vi "MainPannel.vi"() -> ()   [LabVIEW 2018]
uses:
  Controls/StageInfo.ctl
  Controls/GeneratorInfo.ctl
  <vilib>/userdefined/High Color/nirio_resource_hc.ctl
  Controls/DigitizerInfo.ctl
  Controls/AdditionalData.ctl
  <vilib>/Heliosphere Research LLC/Advanced Plotting Toolkit/properties/Colormap_Map.ctl
  <vilib>/Math Plots/3D Math Plots/3D Mesh/3D Mesh XCtrl/3D Mesh.xctl
  Controls/ScanStates.ctl
  Program_Files/Labview2018/MAIN/instr.lib/ASI TG-1000/Public/Utility/Axis Name.ctl
  <vilib>/UPVI/lvhdf5/dataset.llb/LVH5D Operation.ctl
  <extravilib>/ChannelInstances/Tag-c(t'AdditionalData.ctl',bool)/Write With Abort.vi
  <extravilib>/ChannelInstances/Tag-c(t'GeneratorInfo.ctl',bool)/Write With Abort.vi
  <extravilib>/ChannelInstances/Tag-c(t'DigitizerInfo.ctl',bool)/Write With Abort.vi
  <extravilib>/ChannelInstances/Tag-c(t'StageInfo.ctl',bool)/Write With Abort.vi
  <extravilib>/ChannelInstances/Tag-c(t'AdditionalData.ctl',bool)/Read With Abort.vi
  <extravilib>/ChannelInstances/Tag-c(t'GeneratorInfo.ctl',bool)/Read With Abort.vi
  <extravilib>/ChannelInstances/Tag-c(t'DigitizerInfo.ctl',bool)/Read With Abort.vi
  <extravilib>/ChannelInstances/Tag-c(t'StageInfo.ctl',bool)/Read With Abort.vi
  <extravilib>/ChannelInstances/Stream-c(i32,i32,a[.](u64))/Read With Abort.vi
  <extravilib>/ChannelInstances/Stream-c(i32,i32,a[.](u64))/Write With Abort.vi
  <extravilib>/ChannelInstances/Stream-c(i32,i32,a[.](u64))/EndpointRead.vi
  <extravilib>/ChannelInstances/Stream-c(i32,i32,a[.](u64))/Endpoint.vi
  <extravilib>/ChannelInstances/Tag-c(t'DigitizerInfo.ctl',bool)/Instantiate.vi
  <extravilib>/ChannelInstances/Tag-c(t'DigitizerInfo.ctl',bool)/Endpoint.vi
  <extravilib>/ChannelInstances/Tag-c(t'GeneratorInfo.ctl',bool)/Instantiate.vi
  <extravilib>/ChannelInstances/Tag-c(t'GeneratorInfo.ctl',bool)/Endpoint.vi
  <extravilib>/ChannelInstances/Tag-c(t'AdditionalData.ctl',bool)/Instantiate.vi
  <extravilib>/ChannelInstances/Tag-c(t'AdditionalData.ctl',bool)/Endpoint.vi
  <extravilib>/ChannelInstances/Tag-c(t'StageInfo.ctl',bool)/Instantiate.vi
  <extravilib>/ChannelInstances/Tag-c(t'AdditionalData.ctl',bool)/EndpointRead.vi
  <extravilib>/ChannelInstances/Tag-c(t'GeneratorInfo.ctl',bool)/EndpointRead.vi
  <extravilib>/ChannelInstances/Tag-c(t'DigitizerInfo.ctl',bool)/EndpointRead.vi
  <extravilib>/ChannelInstances/Tag-c(t'StageInfo.ctl',bool)/EndpointRead.vi
  <vilib>/UPVI/lvhdf5/dataset.llb/Simple OpenCreateReplace Dataset (Variant).vi
  <extravilib>/ChannelInstances/Stream-c(i32,i32,a[.](u64))/Instantiate.vi
  <extravilib>/ChannelInstances/Stream-c(i32,i32,a[.](u64))/)Channel.vi
  <resource>/ChannelSupport/_ChannelSupport/WaitIfNeeded.vi
  <vilib>/UPVI/lvhdf5/dataset.llb/Append Element(s) to Dataset (Variant).vi
  <vilib>/Math Plots/3D Math Plots/3D Mesh/3D Mesh Datatype/Public/Plot Helper (Vector).vi
  <vilib>/Utility/error.llb/Error Cluster From Error Code.vi
  <vilib>/rvi/errors/niLvFpgaAdjustHostInterfaceError.vi
  <vilib>/FPGAPlugInAG/Dynamic/niLvFpga_Close_Dynamic.vi
  <extravilib>/ChannelInstances/Tag-c(t'StageInfo.ctl',bool)/Endpoint.vi
  <vilib>/UPVI/lvhdf5/dataset.llb/Simple OpenCreateReplace Dataset.xnode
  <vilib>/UPVI/lvhdf5/library.llb/HDF5 Ref.ctl
  <vilib>/UPVI/lvhdf5/dataset.llb/Append Element(s) to Dataset.xnode
  <vilib>/rvi/interface/nirviReadWriteControl/nirviReadWriteControl.xnode
  <vilib>/rvi/interface/nirviCloseFPGA/nirviCloseFPGA.xnode
  <vilib>/rvi/interface/nirviMethod/nirviMethod.xnode
  Program_Files/Labview2018/MAIN/instr.lib/ASI TG-1000/ASI TG-1000.lvlib
  <vilib>/Analysis/NI_AALPro.lvlib
  <vilib>/Math Plots/3D Math Plots/3D Mesh/3D Mesh Datatype/3D Mesh Datatype.lvclass
  <extravilib>/ChannelInstances/Tag-c(t'StageInfo.ctl',bool).lvlib
  <extravilib>/ChannelInstances/Tag-c(t'DigitizerInfo.ctl',bool).lvlib
  <extravilib>/ChannelInstances/Tag-c(t'GeneratorInfo.ctl',bool).lvlib
  <extravilib>/ChannelInstances/Tag-c(t'AdditionalData.ctl',bool).lvlib
  NiFpgaLv.dll
  <vilib>/rvi/interface/Simulation/niFpgaSimulationCallBeginRW.vi
  <vilib>/FPGAPlugInAG/Dynamic/niLvFpga_ReadFifo_Dynamic.vi
  <vilib>/rvi/errors/niLvFpgaMergeErrorWithErrorCode.vi
  <extravilib>/ChannelInstances/Stream-c(i32,i32,a[.](u64)).lvlib
  <vilib>/Heliosphere Research LLC/Advanced Plotting Toolkit/Advanced Plotting Toolkit.lvlib
panel:
  in  "Find Delay after Trig":bool
  in  "Threshold Magnitude":dbl
  out "State":T1
  in  "Setup Scan":bool
  out "Stage Set":bool
  out "Additional Data Set?":bool
  out "3D Mesh":refnum<class "3D Plot Datatype.lvclass">[](xcontrol)
  in  "Data Gating":bool
  in  "Colorbar":bool
  in  "Axis":bool
  in  "Colormap":T2
  out "Image":picture
  in  "Emergercy Stop":bool
  in  "Length":dbl
  in  "Start Depth":dbl
  in  "Pixel/mm":bool=TRUE caption="Mode"
  in  "Z Position":dbl
  in  "Y Position":dbl
  in  "X Position":dbl
  out "Stage Position":cluster{dbl[], dbl[]}(graph) caption="XY Graph - Dark"
  in  "Waveform Tab Control":T3(tab)
  out "Input Graph":cluster{"tv":dbl[], "DAC Codes":u16[]}(graph)
  out "Output Graph":cluster{dbl, dbl, ext[][]}(graph)
  out "Output Graph FFT":cluster{dbl[], dbl[]}(graph)
  out "Additional Info":T4
  in  "Setup Additional Data":bool
  out "Digitizer Info":T5
  out "Default Configured?":bool
  out "Clocking Option Configured?":bool
  out "TIS Configured?":bool
  in  "Setup Digitizer":bool
  out "Generator Info":T7
  out "Stage Setup Info":T8
  in  "Setup Generator":bool
  in  "Setup Stage":bool
  in  "Update Stage Pos":bool
  out "Digitizer Configured?":bool
  out "Generator Ready?":bool
  out "Total Pixels":i32
  out "Stage Setup?":bool
  out "Scan Time":dbl
  out "Y Resolution":dbl
  out "X Resolution":dbl
  in  "Stage Control":T9(tab)
  in  "Stage Port":refnum<visa-resource-name>
  in  "Scan Mode":enum16{"Raster Scan", "Serpentine Scan"}(ring)
  in  "Start X":dbl
  in  "Start Y":dbl
  in  "Stop X":dbl=5.0 caption="X Length (mm)"
  in  "Stop Y":dbl=5.0 caption="Y Length (mm)"
  in  "Overshoot":dbl=1.0
  in  "X Speed (mms)":dbl=1.0
  in  "Y Speed (mms)":dbl=1.0
  in  "X Pixels Count":i32=40
  in  "Y Lines Count":i32=10
  in  "Use Current Position as Start":bool=TRUE caption="Checkbox"
  in  "Generator ID":tag
  in  "Digitizer ID":tag
  in  "Record Size (Samples)":u32=1024
  in  "Delay after Trigger (us)":dbl
  in  "Sampling Rate (Fs)":dbl=400000000.0 format="%#_6p"
  in  "Temperature":dbl
  in  "Trigger Type":enum8{"Software", "Data Edge"}(ring)
  in  "Trigger Level (V)":dbl
  in  "File Directory":path
  in  "Filename":string
  in  "Open Stage Port":bool
  in  "Move Z":i16(knob) scale=0.0..50.0
  in  "Move Y":i16(knob) scale=0.0..50.0
  in  "Move X":i16(knob) scale=0.0..50.0
  in  "Precision":i16(slide) scale=0.0..3.0
  in  "SendCommand To Stage":bool
  in  "Debug Mode":bool
  out "Response":string
  in  "Command":string
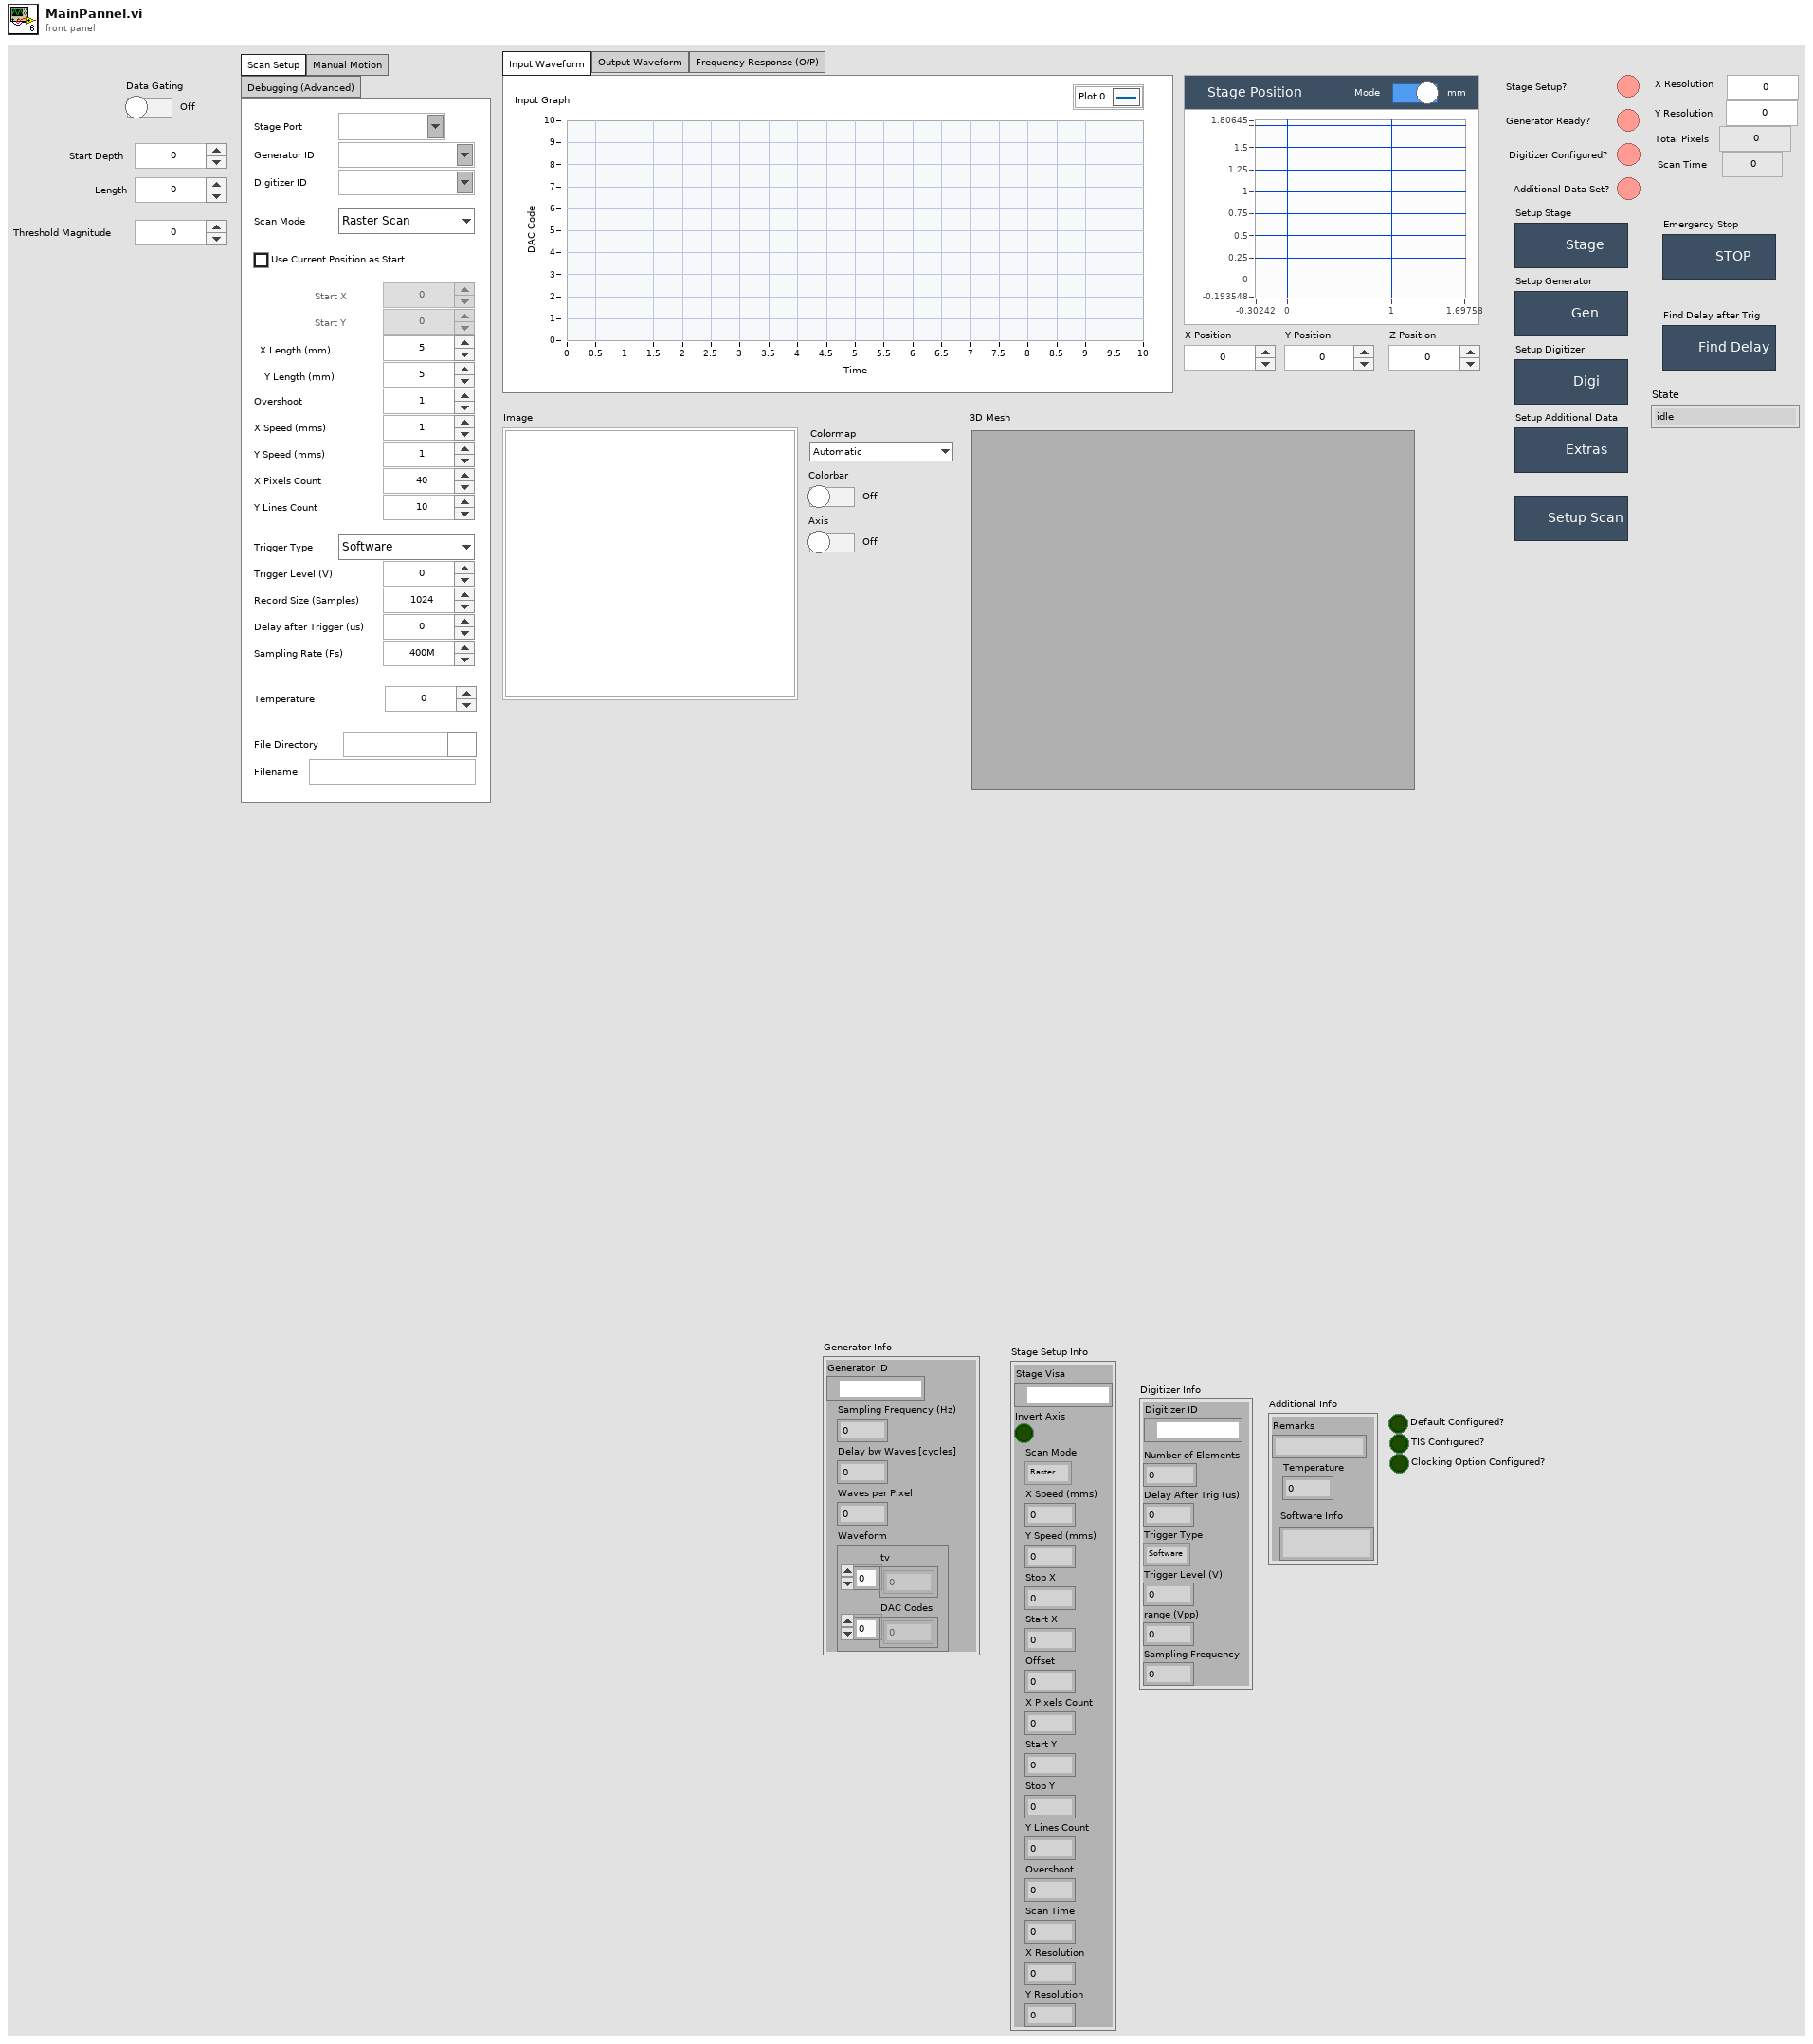
[diagram p1: front panel]
types:
  T1 = typedef "ScanStates.ctl" = enum16{"idle", "init", "scan", "endscan", "closefiles"}
  T2 = typedef "Advanced Plotting Toolkit.lvlib/Colormap_Map.ctl" = enum16{"Automatic", "Rainbow", "Hot and Cold", "White-Black", "White-Blue", "White-Green", "White-Red", "Fire", "Water", "Earth", "Air", "Pastel", "Banded", "Stepped"}
  T3 = enum32{"Input Waveform", "Output Waveform", "Frequency Response (O/P)"}
  T4 = typedef "AdditionalData.ctl" = cluster{"Remarks":string, "Temperature":dbl, "Software Info":string}
  T5 = typedef "DigitizerInfo.ctl" = cluster{"Digitizer ID":T6, "Number of Elements":u16, "Delay After Trig (us)":dbl, "Trigger Type":enum8{"Software", "Data Edge"}, "Trigger Level (V)":dbl, "range (Vpp)":dbl, "Sampling Frequency":dbl}
  T6 = typedef "nirio_resource_hc.ctl" = tag
  T7 = typedef "GeneratorInfo.ctl" = cluster{"Generator ID":T6, "Sampling Frequency (Hz)":u64, "Delay bw Waves [cycles]":u16, "Waves per Pixel":u32, "Waveform":cluster{"tv":dbl[], "DAC Codes":u16[]}}
  T8 = typedef "StageInfo.ctl" = cluster{"Stage Visa":refnum<visa-resource-name>, "Invert Axis":bool, "Scan Mode":enum16{"Raster Scan", "Serpentine Scan"}, "X Speed (mms)":dbl, "Y Speed (mms)":dbl, "Stop X":dbl, "Start X":dbl, "Offset":dbl, "X Pixels Count":i32, "Start Y":dbl, "Stop Y":dbl, "Y Lines Count":i32, "Overshoot":dbl, "Scan Time":dbl, "X Resolution":dbl, "Y Resolution":dbl}
  T9 = enum32{"Scan Setup", "Manual Motion", "Debugging (Advanced)"}
  T10 = enum8{"Enabled", "Disabled", "Disabled and Grayed Out"}
  T11 = typedef "Tag-c(t'StageInfo.ctl',bool).lvlib/))Channel.ctl" = refnum<queue>
  T12 = typedef "ASI TG-1000.lvlib/Axis Name.ctl" = enum8{"undefined", "A", "B", "C", "D", "E", "F", "G", "H", "I", "J", "K", "L", "M", "N", "O", "P", "Q", "R", "S", "T", "U", "V", "W", "X", "Y", "Z"}
  T13 = cluster{"Additional Info":T4, "Additional Data Set?":bool}
  T14 = typedef "Tag-c(t'AdditionalData.ctl',bool).lvlib/))Channel.ctl" = refnum<queue>
  T15 = typedef "Tag-c(t'GeneratorInfo.ctl',bool).lvlib/))Channel.ctl" = refnum<queue>
  T16 = typedef "Tag-c(t'DigitizerInfo.ctl',bool).lvlib/))Channel.ctl" = refnum<queue>
  T17 = typedef "LVH5D Operation.ctl" = enum16{"open", "replace", "create", "open or create", "create or replace", "create or replace with confirmation"}
  T18 = typedef "HDF5 Ref.ctl" = refnum<k1>
  T19 = typedef "Stream-c(i32,i32,a[.](u64)).lvlib/)Channel.ctl" = refnum<queue>
  T20 = cluster{"X Pixel":i32, "Y Pixel":i32, "Data":u64[]}
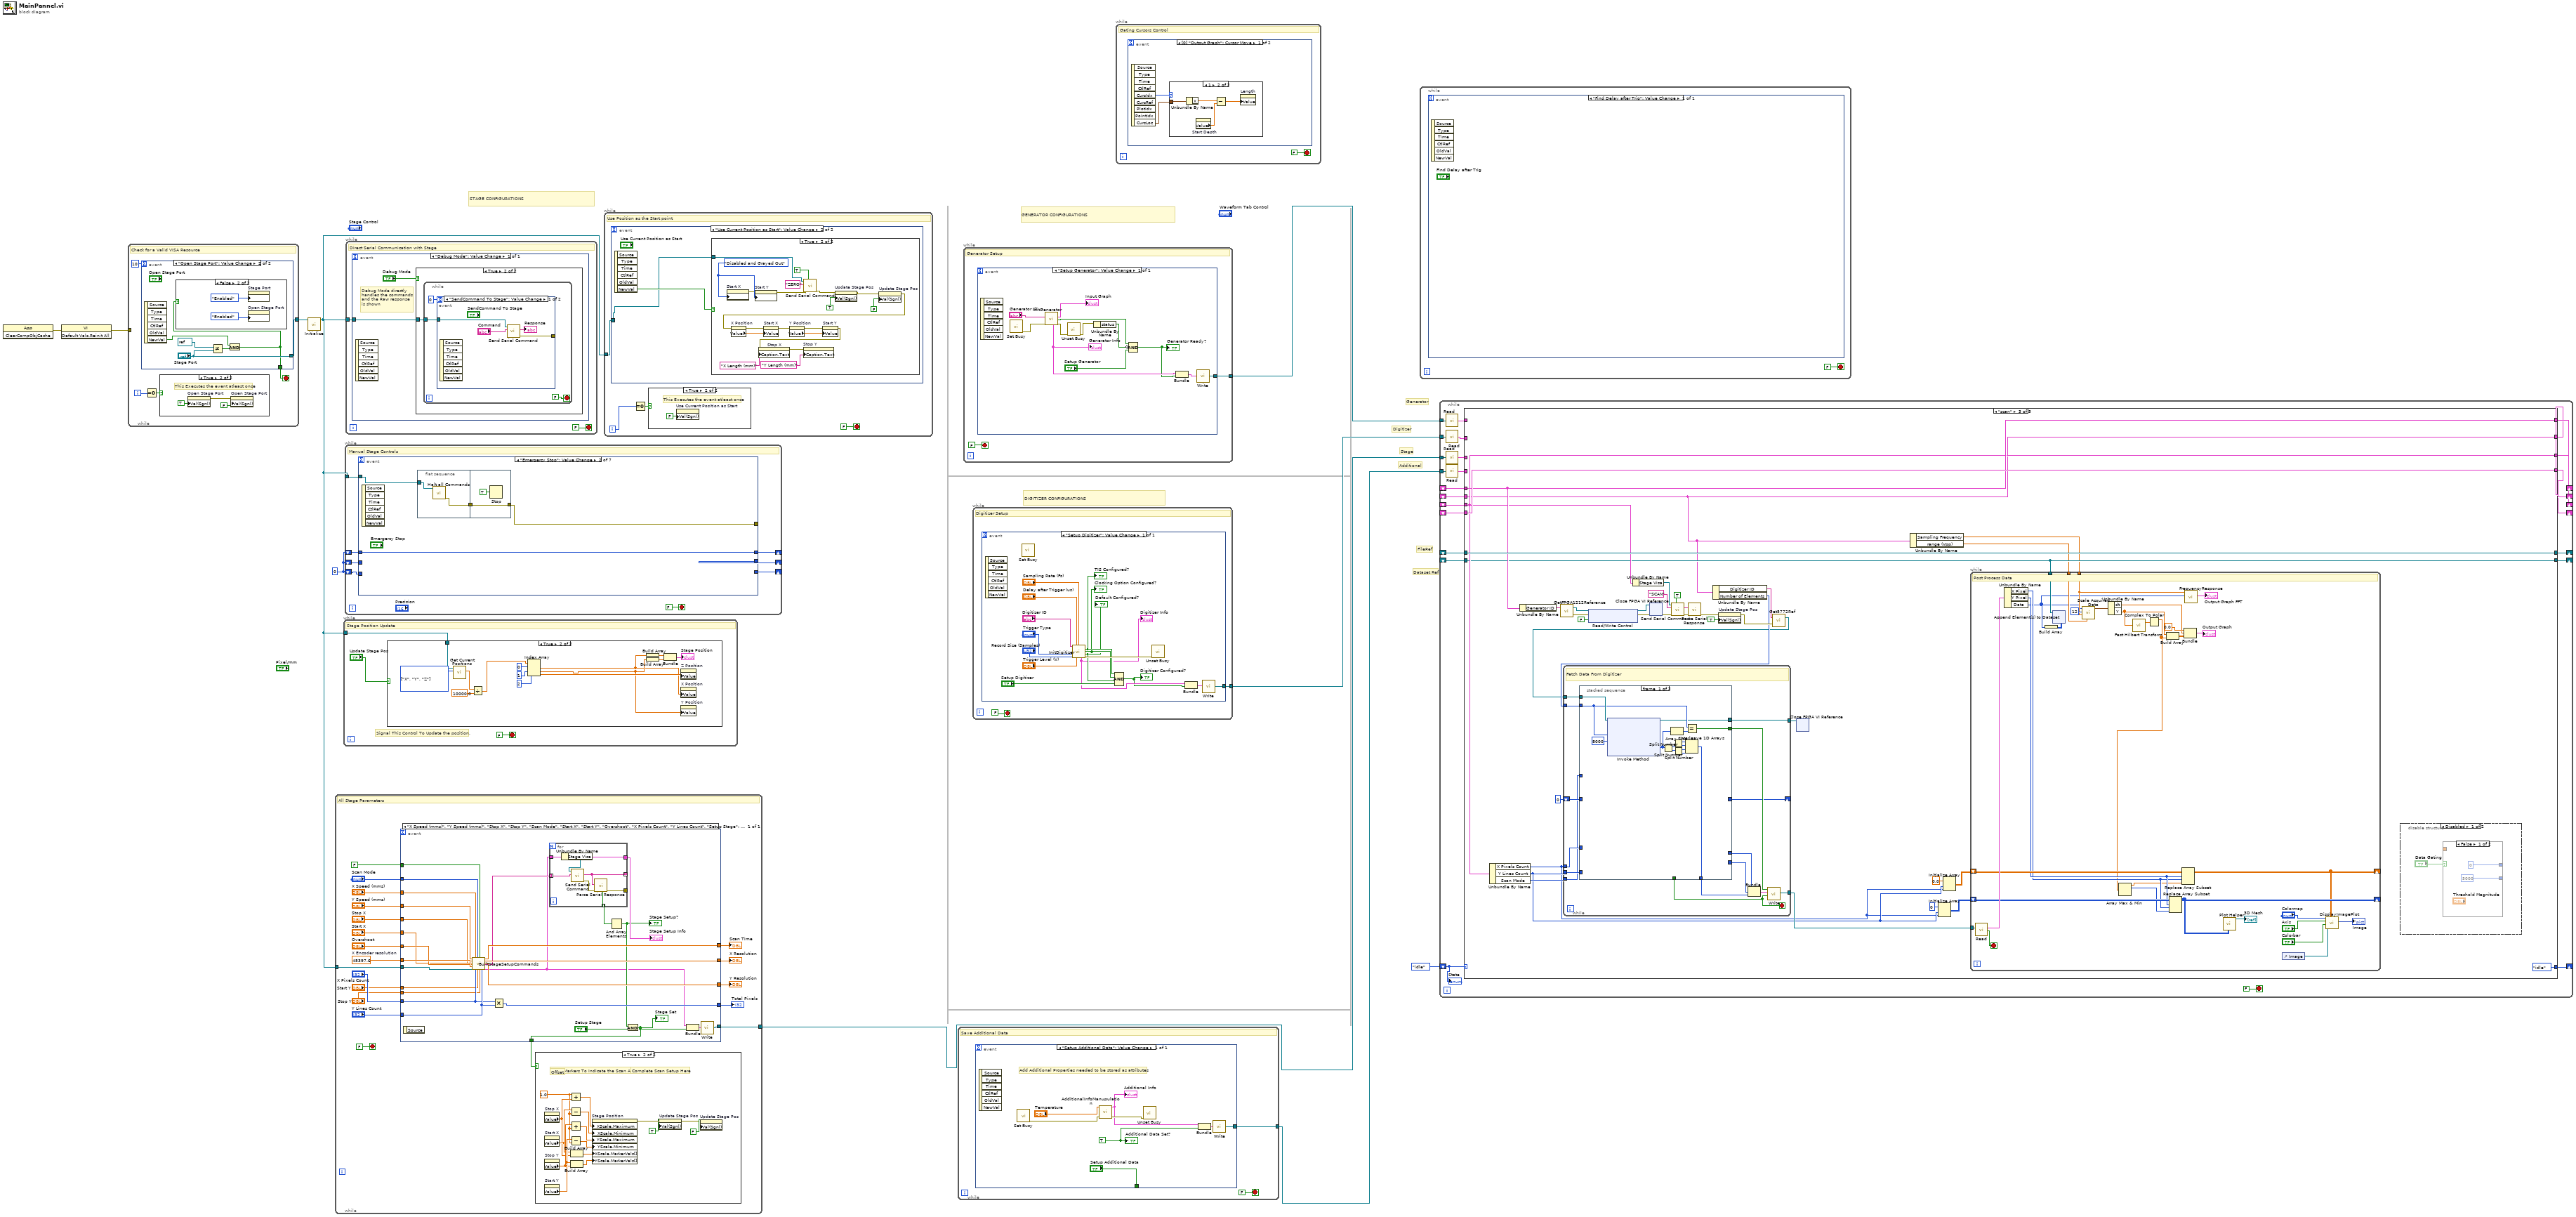
[diagram p0: block diagram]
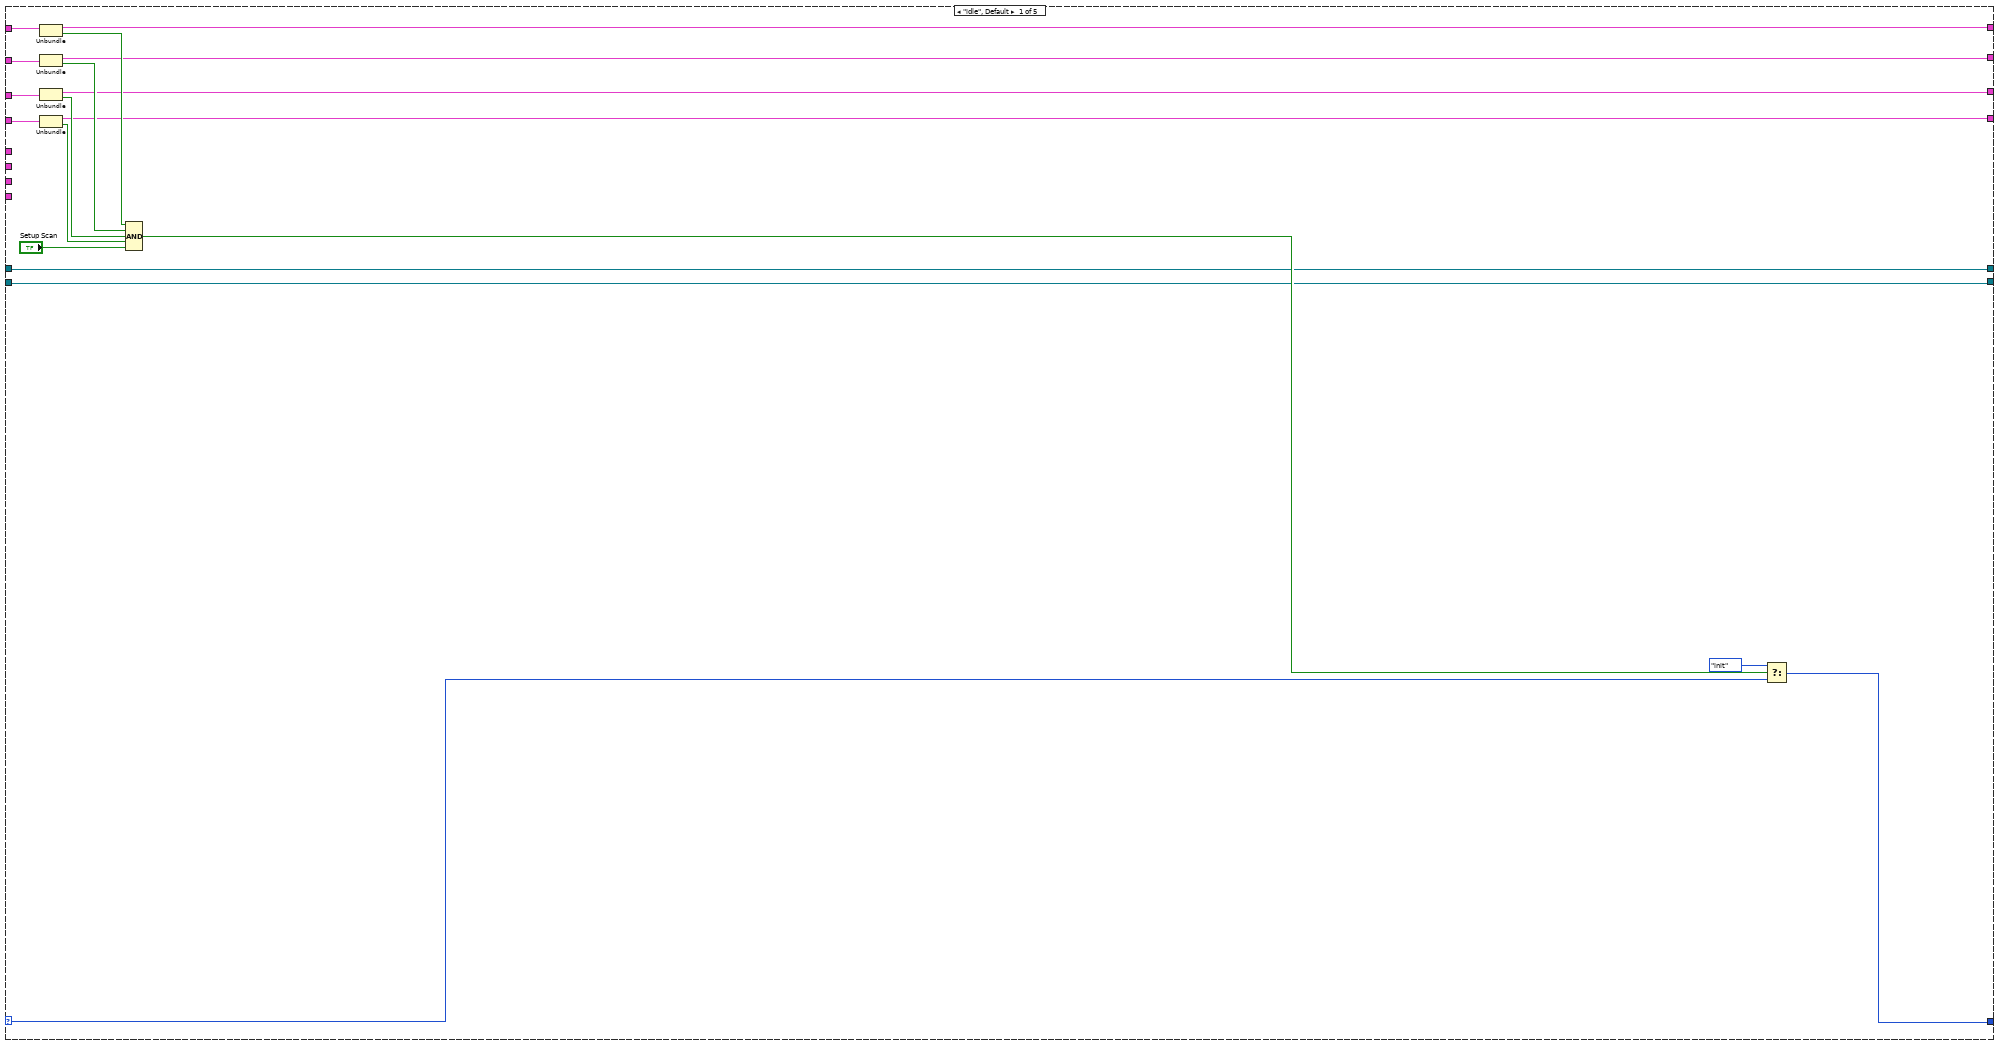
[diagram p2: hidden frame]
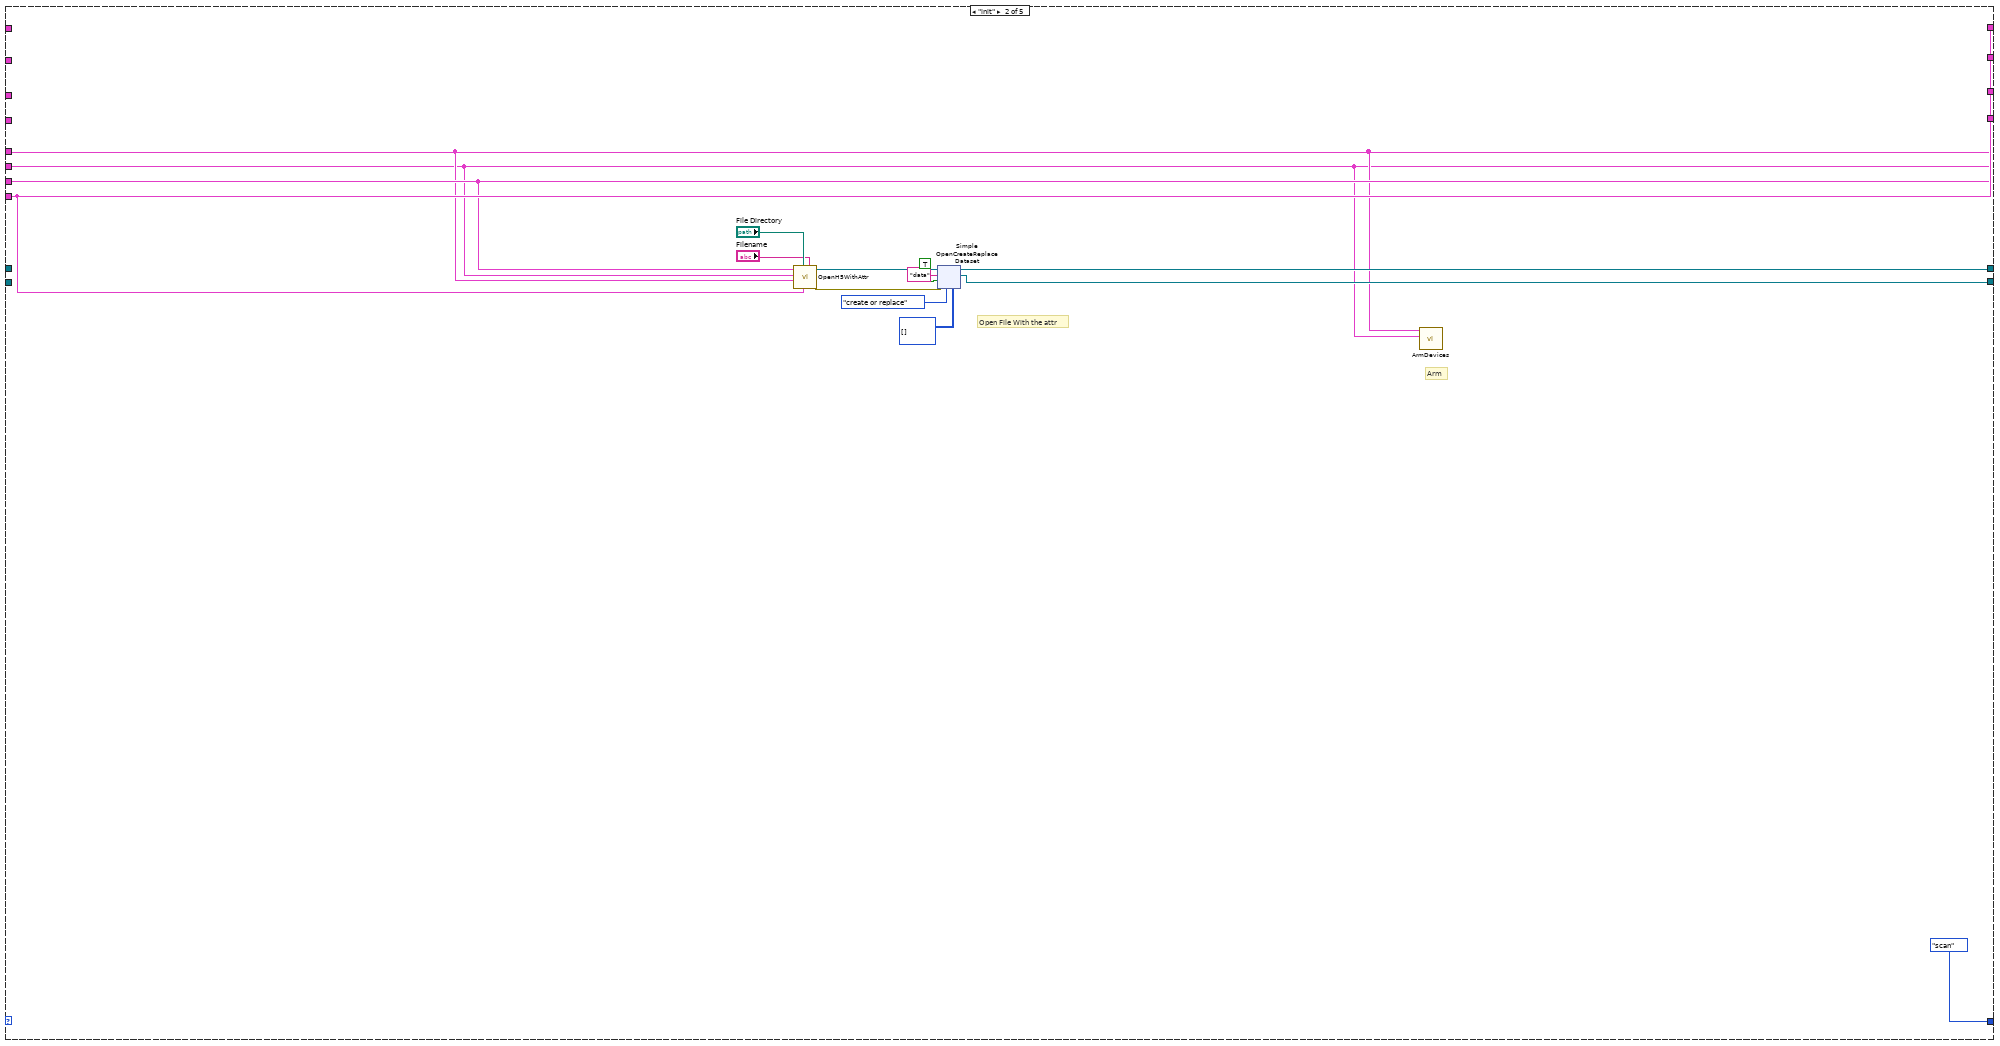
[diagram p3: hidden frame]
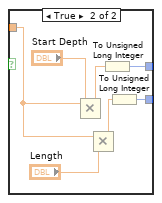
[diagram p4: hidden frame]
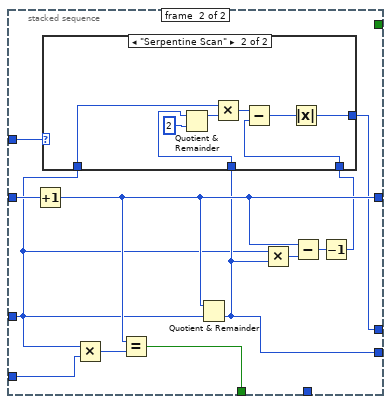
[diagram p6: hidden frame]
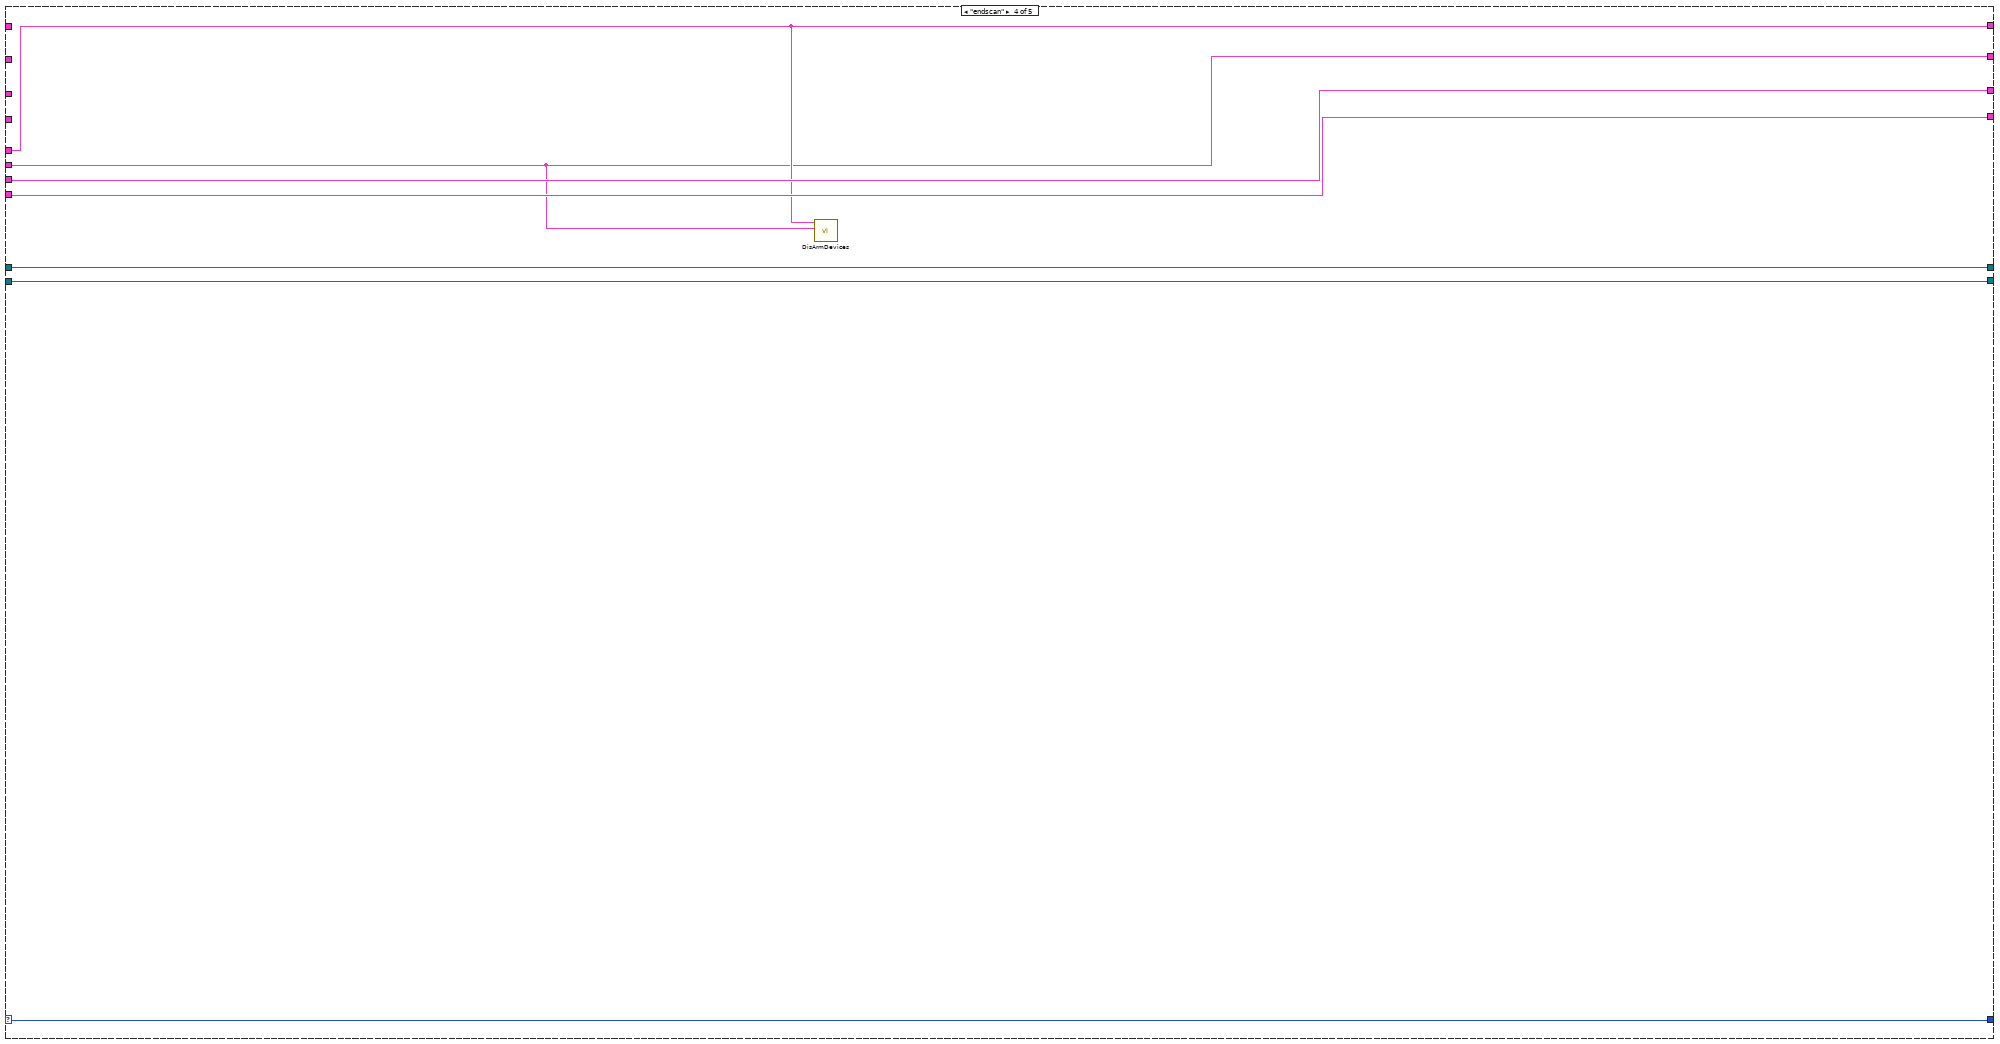
[diagram p8: hidden frame]
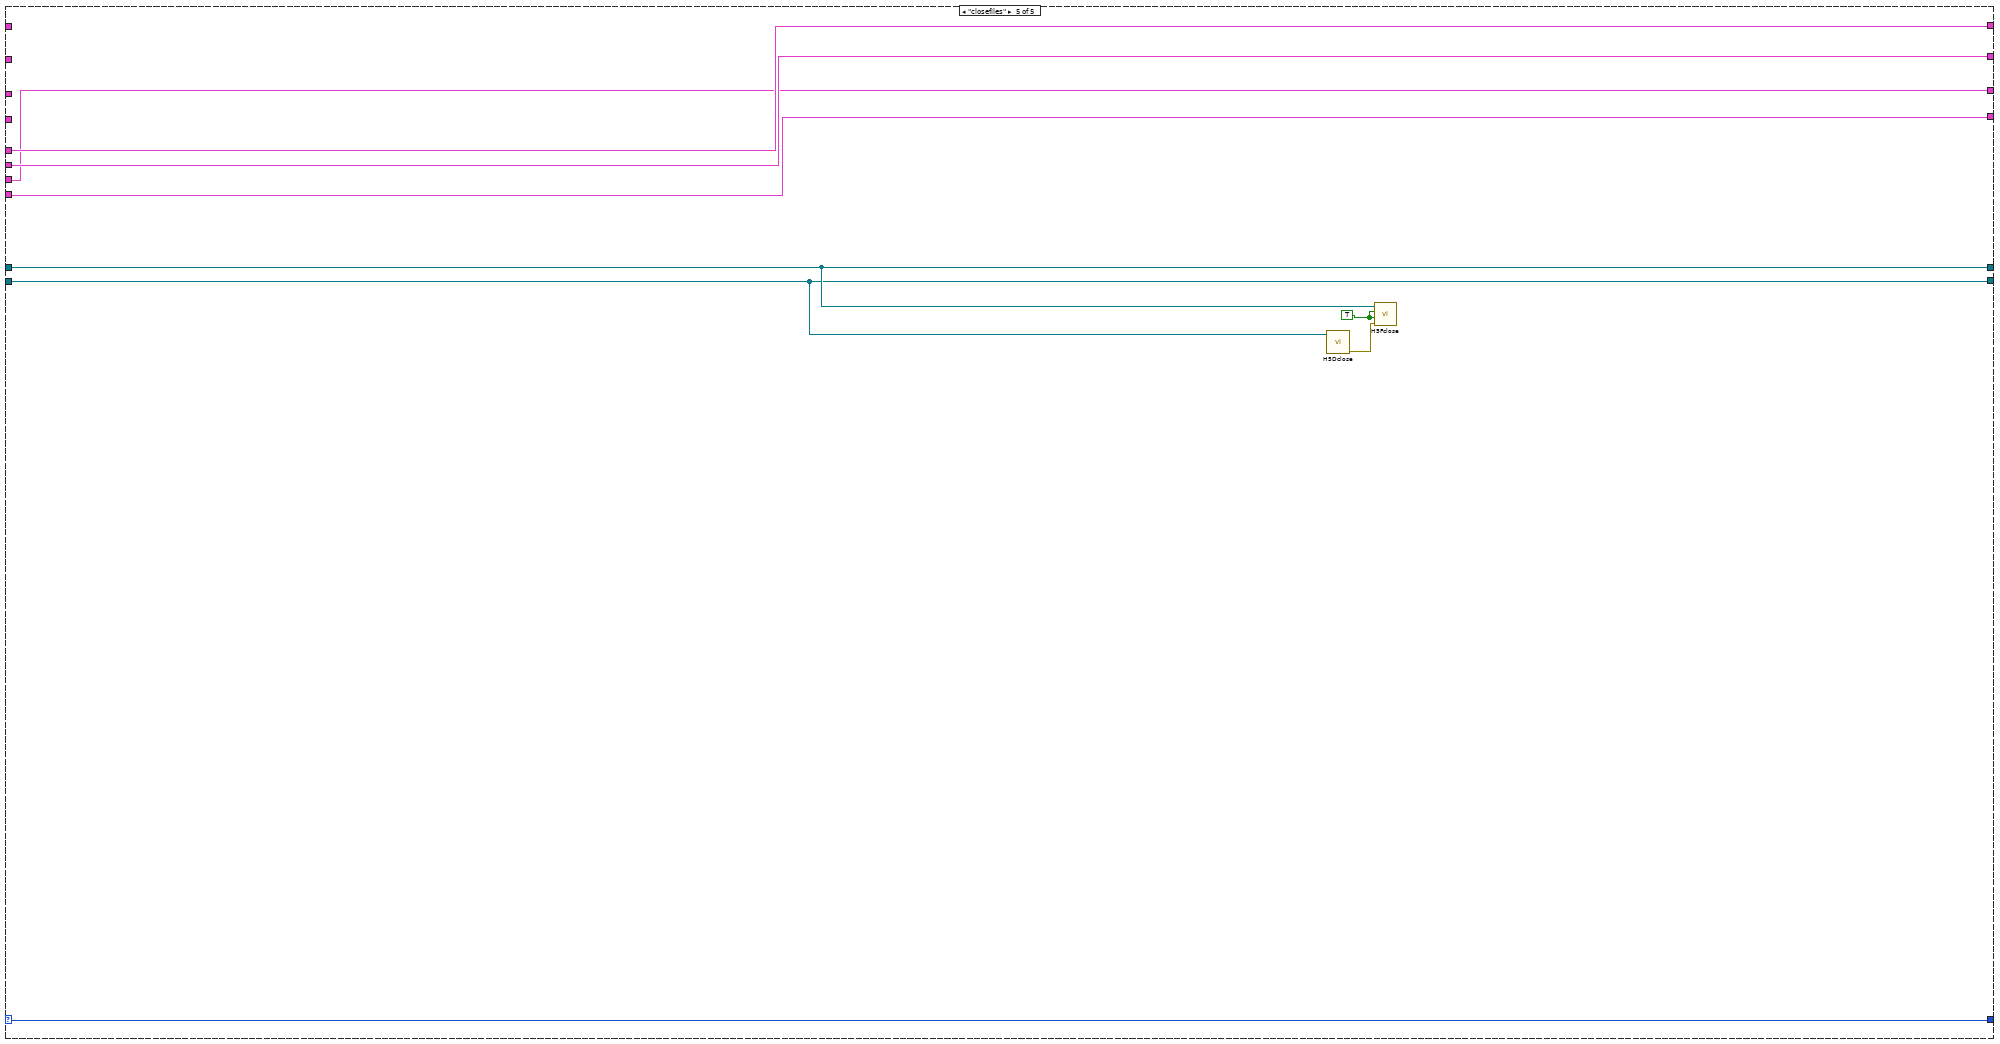
[diagram p9: hidden frame]
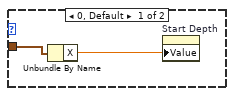
[diagram p10: hidden frame]
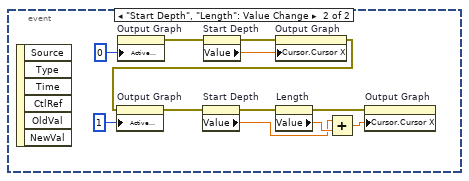
[diagram p11: hidden frame]
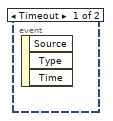
[diagram p14: hidden frame]
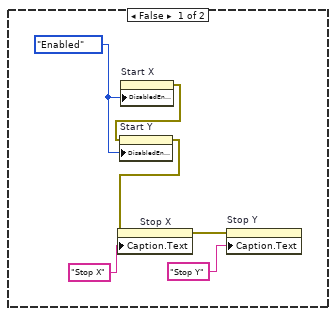
[diagram p15: hidden frame]
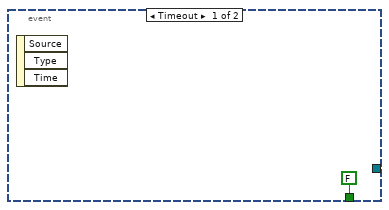
[diagram p17: hidden frame]
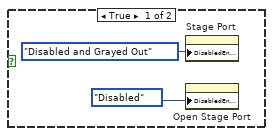
[diagram p18: hidden frame]
diagram:
  w10 = 0
  # "Dataset Ref"
  # "FileRef"
  # "Additional"
  # "Stage"
  # "Digitizer"
  # "Generator"
  # "DIGITIZER CONFIGURATIONS"
  # "GENERATOR CONFIGURATIONS"
  # "STAGE CONFIGURATIONS"
  n1 = invoke class="App" method="ClearCompObjCache"() -> (error out=w4:errorcluster)  [unwired: 3 in, 2 out]
  n2 = invoke class="VI" method="Default Vals.Reinit All"(error in=w4) -> (error out=w3:errorcluster)  [unwired: 2 in, 2 out]
  n3 = while {
    tunnel: [w14] -> w9
    tunnel: w3 -> [_]
    i -> [w11]
    stop <- w13 stop-if-true
    # "Check for a Valid VISA Resource"
    n4 = event shown="[1] \"Open Stage Port\": Value Change" {
      selector: _ -> [_ _]
      dyn-events: _ -> [_ _]
      timeout: 10 -> [_ _]
      tunnel: [_ "Stage Port"] -> w14
      tunnel: [FALSE w20] -> w13
      event Timeout {
        n5 = event-data() -> ()  [unwired: 1 in, 3 out]
      }
      event "Open Stage Port": Value Change {
        n6 = event-data() -> ("NewVal"=w21:bool)  [unwired: 1 in, 5 out]
        n7 = Not Equal?(x=refnum<visa-resource-name> refnum, y="Stage Port") -> (x != y?=w22:bool)
        n8 = And(x=w21, y=w22) -> (x .and. y?=w20:bool)
        n9 = case shown="False" w20 {
          frame True {
            n10 = property on="Stage Port" class="VISAName"("DisabledEnum"=T10."Disabled and Grayed Out" ("Disabled")) -> ()  [unwired: 2 in, 2 out]
            n11 = property on="Open Stage Port" class="Bool (strict)"("DisabledEnum"=T10."Disabled" ("Disabled")) -> ()  [unwired: 2 in, 2 out]
          }
          frame False {
            n12 = property on="Stage Port" class="VISAName"("DisabledEnum"=T10."Enabled" ("Disabled")) -> ()  [unwired: 2 in, 2 out]
            n13 = property on="Open Stage Port" class="Bool (strict)"("DisabledEnum"=T10."Enabled" ("Disabled")) -> ()  [unwired: 2 in, 2 out]
          }
        }
      }
    }
    n14 = Equal To 0?(x=w11) -> (x = 0?=w12:bool)
    n15 = case shown="True" w12 {
      frame False {
      }
      frame True {
        # "This Executes the event atleast once"
        n16 = property on="Open Stage Port" class="Bool (strict)"("Val(Sgnl)"=TRUE ("Value (Signaling)")) -> (error out=w16:errorcluster)  [unwired: 2 in, 1 out]
        n17 = property on="Open Stage Port" class="Bool (strict)"(error in=w16, "Val(Sgnl)"=FALSE ("Value (Signaling)")) -> ()  [unwired: 1 in, 2 out]
      }
    }
  }
  n18 = call "Initialize.vi"("VISA resource name"=w9) -> ("VISA resource name out"=w5:refnum<visa-resource-name>)  [unwired: 9 in, 1 out]
  n19 = while {
    tunnel: w5 -> [w48]
    tunnel: [w29] -> w8
    stop <- FALSE stop-if-true
    w44 = 45397.6  # X Encoder resolution
    # "All Stage Parameters"
    n20 = event shown="[0] \"X Speed (mms)\", \"Y Speed (mms)\", \"Stop X\", \"Stop Y\", \"Scan Mode\", \"Start X\", \"Start Y\", \"Overshoot\", \"X Pixels Count\", \"Y Lines Count\", \"Setup Stage\": Value Change" {
      selector: _ -> [_]
      dyn-events: _ -> [_]
      timeout: _ -> [_]
      tunnel: w48 -> [w89]
      tunnel: FALSE -> [w88]
      tunnel: "Y Lines Count" -> [w87]
      tunnel: "X Pixels Count" -> [w86]
      tunnel: w44 -> [w85]
      tunnel: "Y Speed (mms)" -> [w84]
      tunnel: "Scan Mode" -> [w83]
      tunnel: "Overshoot" -> [w82]
      tunnel: "Stop Y" -> [w81]
      tunnel: "Stop X" -> [w80]
      tunnel: "Start Y" -> [w79]
      tunnel: "Start X" -> [w78]
      tunnel: "X Speed (mms)" -> [w77]
      tunnel: [w76] -> w35
      tunnel: [w75] -> w34
      tunnel: [w74] -> w33
      tunnel: [w73] -> w32
      tunnel: [w66] -> w30
      tunnel: [w64] -> w29
      event "X Speed (mms)", "Y Speed (mms)", "Stop X", "Stop Y", "Scan Mode", "Start X", "Start Y", "Overshoot", "X Pixels Count", "Y Lines Count", "Setup Stage": Value Change {
        n21 = event-data() -> ()  [unwired: 1 in, 1 out]
        n22 = call "BuiltStageSetupCommands.vi"("Y Speed (mms)"=w84, "Stop X"=w80, "Start X"=w78, "Overshoot"=w82, "X Encoder resolution"=w85, "Stage Visa"=w89, "X Speed (mms)"=w77, "X Pixels Count"=w86, "Scan Mode"=w83, "Start Y"=w79, "Invert Axis"=w88, "Stop Y"=w81, "Y Lines Count"=w87) -> ("Scan Time"=w75:dbl, "X resolution"=w73:dbl, "Y Resolution"=w74:dbl, "Commands array"=w70:string[], "Stage Setup Info"=w67:T8)  [unwired: 2 in]
        n23 = Multiply(x=w86, y=w87) -> (x*y=w76:i32)
        n24 = for {
          tunnel: w70 -> [w96] mode=indexing
          tunnel: [w95] -> _ mode=indexing
          tunnel: [w93] -> w71 mode=indexing
          tunnel: [w92] -> _
          tunnel: w67 -> [w90]
          tunnel: [w90] -> w72
          n25 = Unbundle By Name(w90) -> ("Stage Visa"=w91:refnum<visa-resource-name>)
          n26 = call "Send Serial Command.vi"("Command"=w96, "VISA in"=w91) -> ("error out"=w94:errorcluster, "Response"=w95:string)  [unwired: 7 in, 1 out]
          n27 = call "Parse Serial Response.vi"("error in (no error)"=w94, "Raw Response"=w95) -> ("error out"=w92:errorcluster, "As expected?"=w93:bool)  [unwired: 6 in, 2 out]
        }
        "Stage Setup Info" <- w72
        n28 = And Array Elements(Boolean array=w71) -> (logical AND=w69:bool)
        "Stage Setup?" <- w69
        n29 = And(x=w69, y="Setup Stage") -> (x .and. y?=w66:bool)
        "Stage Set" <- w66
        n30 = Bundle("Stage Setup Info"=w67, w66) -> (w65:cluster{"Stage Setup Info":T8, bool})  [unwired: 1 in]
        n31 = call <extravilib>:"Write.vi"("element"=w65) -> ("channel"=w64:T11)  [unwired: 1 out]
      }
    }
    "X Resolution" <- w32
    "Y Resolution" <- w33
    "Scan Time" <- w34
    "Total Pixels" <- w35
    n32 = case shown="True" w30 {
      frame False {
      }
      frame True {
        w51 = 1.0 ("y")
        # "Complete Scan Setup Here"
        # "Draw Markers To Indicate the Scan Area"
        # "Offset"
        n33 = property on="Stop X" class="DigNum (strict)"() -> ("Value"=w59:dbl)  [unwired: 2 in, 2 out]
        n34 = property on="Start X" class="DigNum (strict)"() -> ("Value"=w60:dbl)  [unwired: 2 in, 2 out]
        n35 = property on="Stop Y" class="DigNum (strict)"() -> ("Value"=w62:dbl)  [unwired: 2 in, 2 out]
        n36 = property on="Start Y" class="DigNum (strict)"() -> ("Value"=w63:dbl)  [unwired: 2 in, 2 out]
        n37 = Add(x=w51, y=w59) -> (x+y=w57:dbl)
        n38 = Subtract(x=w60, y=w51) -> (x-y=w56:dbl)
        n39 = Add(x=w62, y=w51) -> (x+y=w58:dbl)
        n40 = Subtract(x=w63, y=w51) -> (x-y=w61:dbl)
        n41 = Build Array(w60, w59) -> (w54:dbl[])
        n42 = Build Array(w63, w62) -> (w55:dbl[])
        n43 = property on="Stage Position" class="XYGraph (strict)"("XScale.Maximum"=w57, "XScale.Minimum"=w56, "YScale.Maximum"=w58, "YScale.Minimum"=w61, "XScale.MarkerVals[]"=w54, "YScale.MarkerVals[]"=w55) -> (error out=w53:errorcluster)  [unwired: 2 in, 1 out]
        n44 = property on="Update Stage Pos" class="Bool (strict)"(error in=w53, "Val(Sgnl)"=TRUE ("Value (Signaling)")) -> (error out=w49:errorcluster)  [unwired: 1 in, 1 out]
        n45 = property on="Update Stage Pos" class="Bool (strict)"(error in=w49, "Val(Sgnl)"=FALSE ("Value (Signaling)")) -> ()  [unwired: 1 in, 2 out]
      }
    }
  }
  n46 = while {
    tunnel: w5 -> [w98]
    stop <- FALSE stop-if-true
    # "Signal This Control To Update the position."
    # "Stage Position Update"
    n47 = case shown="True" "Update Stage Pos" {
      tunnel: w98 -> [_ w113]
      frame False {
      }
      frame True {
        w110 = T12[] [enum."X", enum."Y", enum."Z"] items=["undefined", "A", "B", "C", "D", "E", "F", "G", "H", "I", "J", "K", "L", "M", "N", "O", "P", "Q", "R", "S", "T", "U", "V", "W", "X", "Y", "Z"] ("Array of axes")
        n48 = call "Get Current Positions.vi"("Array of axes"=w110, "VISA in"=w113) -> ("Array of positions [internal units]"=w112:dbl[])  [unwired: 7 in, 2 out]
        n49 = Divide(x=w112, y=10000.0) -> (x/y=w102:dbl[])
        n50 = Index Array(array=w102, index #1=0 ("index"), index #2=1 ("index"), index #3=2 ("index")) -> (element #1=w100:dbl, element #2=w101:dbl, element #3=w107:dbl)
        n51 = Build Array(w100) -> (w109:dbl[])
        n52 = Build Array(w101) -> (w108:dbl[])
        n53 = Bundle(w109, w108) -> (→"Stage Position":cluster{dbl[], dbl[]})  [unwired: 1 in]
        n54 = property on="Z Position" class="DigNum (strict)"("Value"=w107) -> ()  [unwired: 2 in, 2 out]
        n55 = property on="X Position" class="DigNum (strict)"("Value"=w100) -> ()  [unwired: 2 in, 2 out]
        n56 = property on="Y Position" class="DigNum (strict)"("Value"=w101) -> ()  [unwired: 2 in, 2 out]
      }
    }
  }
  n57 = while {
    shift-right: [w120] -> _
    shift-left: w10 -> [w121]
    tunnel: w5 -> [w118]
    shift-right: [w117] -> _
    shift-left: w10 -> [w114]
    shift-right: [w116] -> _
    shift-left: w10 -> [w115]
    stop <- FALSE stop-if-true
    # "Manual Stage Controls"
    n58 = event shown="[1] \"Emergercy Stop\": Value Change" {
      selector: _ -> [_ _ _ _ _ _ _]
      dyn-events: _ -> [_ _ _ _ _ _ _]
      timeout: _ -> [_ _ _ _ _ _ _]
      tunnel: w121 -> [w139 _ _ _ _ _ _]
      tunnel: [w138 _ _ _ _ _ _] -> w120
      tunnel: w118 -> [w127 w156 w166 w200 w234 w247 w260]
      tunnel: [w122 w155 w161 w192 w225 w238 w251] -> _
      tunnel: [_ _ w172 _ _ _ _] -> w117
      tunnel: w115 -> [_ w154 _ w204 _ _ _]
      tunnel: [_ w154 _ w203 _ _ _] -> w116
      tunnel: w114 -> [_ _ w171 _ _ _ _]
      event "Move X": Value Change {
        # "This Creates a Jogwheel.\nWe can change the range for \nthis if required."
        n59 = event-data() -> ("NewVal"=w144:i16)  [unwired: 1 in, 5 out]
        n60 = property on="Move X" class="Knob (strict)"() -> ("Scale.Maximum"=w141:dbl)  [unwired: 2 in, 2 out]
        n61 = property on="Move X" class="Knob (strict)"() -> ("Scale.Minimum"=w140:dbl)  [unwired: 2 in, 2 out]
        n62 = case shown="Default" w144 {
          selector: w144 -> [w146 _ _]
          tunnel: w141 -> [_ w149 _]
          tunnel: w140 -> [_ _ w152]
          tunnel: [w146 w149 w152] -> w143
          tunnel: [w145 w148 w150] -> w138
          tunnel: w139 -> [w145 w147 w151]
          frame Default {
          }
          frame 0 {
            n63 = property on="Move X" class="Knob (strict)"("Value"=w149) -> ()  [unwired: 2 in, 2 out]
            n64 = Decrement(x=w147) -> (x-1=w148:i32)
          }
          frame 50 {
            n65 = property on="Move X" class="Knob (strict)"("Value"=w152) -> ()  [unwired: 2 in, 2 out]
            n66 = Increment(x=w151) -> (x+1=w150:i32)
          }
        }
        n67 = Multiply(x=w141, y=w138) -> (x*y=w142:dbl)
        n68 = property on="Precision" class="Slide (strict)"() -> ("Value"=w137:i16)  [unwired: 2 in, 2 out]
        n69 = Add(x=w143, y=w142) -> (x+y=w132:dbl)
        n70 = Power Of 10(x=w137) -> (10^x=w134:dbl)
        n71 = feedback #1(0.0) -> (w135:dbl)
        n72 = Subtract(x=w132, y=w135) -> (x-y=w136:dbl)
        n73 = feedback-in #1(w132) -> ()
        n74 = Divide(x=w136, y=w134) -> (x/y=w130:dbl)
        n75 = Multiply(x=w130, y=10000.0 ("x")) -> (x*y=w129:dbl)
        n76 = call "Move Axis Relative.vi"("Relative Position [internal units]"=w129, "Axis"=Axis_Name."X", "VISA in"=w127) -> ("error out"=w125:errorcluster)  [unwired: 6 in, 1 out]
        n77 = property on="Update Stage Pos" class="Bool (strict)"(error in=w125, "Val(Sgnl)"=TRUE ("Value (Signaling)")) -> (error out=w123:errorcluster)  [unwired: 1 in, 1 out]
        n78 = property on="Update Stage Pos" class="Bool (strict)"(error in=w123, "Val(Sgnl)"=FALSE ("Value (Signaling)")) -> (error out=w122:errorcluster)  [unwired: 1 in, 1 out]
      }
      event "Emergercy Stop": Value Change {
        n79 = event-data() -> ()  [unwired: 1 in, 6 out]
        n80 = flat-sequence {
          tunnel: w156 -> [w158]
          tunnel: [w157] -> w153
          tunnel: [w160] -> w155
          tunnel: w153 -> [w160]
          frame #0 {
            n81 = call "Halt all Commands.vi"("VISA in"=w158) -> ("error out"=w157:errorcluster)  [unwired: 8 in, 1 out]
          }
          frame #1 {
            n82 = Stop(stop? (T)=TRUE) -> ()
          }
        }
      }
      event "Move Y": Value Change {
        # "This Creates a Jogwheel.\nWe can change the range for \nthis if required."
        n83 = event-data() -> ("NewVal"=w183:i16)  [unwired: 1 in, 5 out]
        n84 = property on="Move Y" class="Knob (strict)"() -> ("Scale.Maximum"=w180:dbl)  [unwired: 2 in, 2 out]
        n85 = property on="Move Y" class="Knob (strict)"() -> ("Scale.Minimum"=w179:dbl)  [unwired: 2 in, 2 out]
        n86 = case shown="Default" w183 {
          selector: w183 -> [w185 _ _]
          tunnel: w180 -> [_ w188 _]
          tunnel: w179 -> [_ _ w191]
          tunnel: [w185 w188 w191] -> w182
          tunnel: [w184 w187 w189] -> w172
          tunnel: w171 -> [w184 w186 w190]
          frame Default {
          }
          frame 0 {
            n87 = Decrement(x=w186) -> (x-1=w187:i32)
          }
          frame 50 {
            n88 = Increment(x=w190) -> (x+1=w189:i32)
          }
        }
        n89 = Multiply(x=w180, y=w172) -> (x*y=w181:dbl)
        n90 = property on="Precision" class="Slide (strict)"() -> ("Value"=w178:i16)  [unwired: 2 in, 2 out]
        n91 = Add(x=w182, y=w181) -> (x+y=w173:dbl)
        n92 = Power Of 10(x=w178) -> (10^x=w175:dbl)
        n93 = feedback #2(0.0) -> (w176:dbl)
        n94 = Subtract(x=w173, y=w176) -> (x-y=w177:dbl)
        n95 = feedback-in #2(w173) -> ()
        n96 = Divide(x=w177, y=w175) -> (x/y=w169:dbl)
        n97 = Multiply(x=w169, y=10000.0 ("x")) -> (x*y=w167:dbl)
        n98 = call "Move Axis Relative.vi"("Relative Position [internal units]"=w167, "Axis"=Axis_Name."Y", "VISA in"=w166) -> ("error out"=w164:errorcluster)  [unwired: 6 in, 1 out]
        n99 = property on="Update Stage Pos" class="Bool (strict)"(error in=w164, "Val(Sgnl)"=TRUE ("Value (Signaling)")) -> (error out=w162:errorcluster)  [unwired: 1 in, 1 out]
        n100 = property on="Update Stage Pos" class="Bool (strict)"(error in=w162, "Val(Sgnl)"=FALSE ("Value (Signaling)")) -> (error out=w161:errorcluster)  [unwired: 1 in, 1 out]
      }
      event "Move Z": Value Change {
        # "This Creates a Jogwheel.\nWe can change the range for \nthis if required."
        n101 = event-data() -> ("NewVal"=w216:i16)  [unwired: 1 in, 5 out]
        n102 = property on="Move Z" class="Knob (strict)"() -> ("Scale.Maximum"=w213:dbl)  [unwired: 2 in, 2 out]
        n103 = property on="Move Z" class="Knob (strict)"() -> ("Scale.Minimum"=w212:dbl)  [unwired: 2 in, 2 out]
        n104 = case shown="Default" w216 {
          selector: w216 -> [w218 _ _]
          tunnel: w213 -> [_ w221 _]
          tunnel: w212 -> [_ _ w224]
          tunnel: [w218 w221 w224] -> w215
          tunnel: [w217 w220 w222] -> w203
          tunnel: w204 -> [w217 w219 w223]
          frame Default {
          }
          frame 0 {
            n105 = Decrement(x=w219) -> (x-1=w220:i32)
          }
          frame 50 {
            n106 = Increment(x=w223) -> (x+1=w222:i32)
          }
        }
        n107 = Multiply(x=w213, y=w203) -> (x*y=w214:dbl)
        n108 = property on="Precision" class="Slide (strict)"() -> ("Value"=w211:i16)  [unwired: 2 in, 2 out]
        n109 = Add(x=w215, y=w214) -> (x+y=w205:dbl)
        n110 = Power Of 10(x=w211) -> (10^x=w208:dbl)
        n111 = feedback #3(0.0) -> (w209:dbl)
        n112 = Subtract(x=w205, y=w209) -> (x-y=w210:dbl)
        n113 = feedback-in #3(w205) -> ()
        n114 = Divide(x=w210, y=w208) -> (x/y=w196:dbl)
        n115 = Divide(x=w196, y=0.254) -> (x/y=w197:dbl)
        n116 = Multiply(x=w197, y=1000.0 ("x")) -> (x*y=w201:dbl)
        n117 = call "Move Axis Relative.vi"("Relative Position [internal units]"=w201, "Axis"=Axis_Name."Z", "VISA in"=w200) -> ("error out"=w198:errorcluster)  [unwired: 6 in, 1 out]
        n118 = property on="Update Stage Pos" class="Bool (strict)"(error in=w198, "Val(Sgnl)"=TRUE ("Value (Signaling)")) -> (error out=w193:errorcluster)  [unwired: 1 in, 1 out]
        n119 = property on="Update Stage Pos" class="Bool (strict)"(error in=w193, "Val(Sgnl)"=TRUE ("Value (Signaling)")) -> (error out=w192:errorcluster)  [unwired: 1 in, 1 out]
      }
      event "X Position": Value Change {
        n120 = event-data() -> ("NewVal"=w237:dbl)  [unwired: 1 in, 5 out]
        n121 = In Range and Coerce(upper limit=110.0, x=w237, lower limit=0.0) -> (coerced(x)=w233:dbl)  [unwired: 1 out]
        n122 = Multiply(x=10000.0, y=w233) -> (x*y=w232:dbl)
        n123 = call "Move Axis to Position.vi"("Position [internal units]"=w232, "Axis"=Axis_Name."X", "VISA in"=w234) -> ("error out"=w228:errorcluster)  [unwired: 6 in, 1 out]
        n124 = property on="Update Stage Pos" class="Bool (strict)"(error in=w228, "Val(Sgnl)"=TRUE ("Value (Signaling)")) -> (error out=w226:errorcluster)  [unwired: 1 in, 1 out]
        n125 = property on="Update Stage Pos" class="Bool (strict)"(error in=w226, "Val(Sgnl)"=FALSE ("Value (Signaling)")) -> (error out=w225:errorcluster)  [unwired: 1 in, 1 out]
      }
      event "Y Position": Value Change {
        n126 = event-data() -> ("NewVal"=w250:dbl)  [unwired: 1 in, 5 out]
        n127 = In Range and Coerce(upper limit=110.0, x=w250, lower limit=0.0) -> (coerced(x)=w246:dbl)  [unwired: 1 out]
        n128 = Multiply(x=10000.0, y=w246) -> (x*y=w245:dbl)
        n129 = call "Move Axis to Position.vi"("Position [internal units]"=w245, "Axis"=Axis_Name."Y", "VISA in"=w247) -> ("error out"=w241:errorcluster)  [unwired: 6 in, 1 out]
        n130 = property on="Update Stage Pos" class="Bool (strict)"(error in=w241, "Val(Sgnl)"=TRUE ("Value (Signaling)")) -> (error out=w239:errorcluster)  [unwired: 1 in, 1 out]
        n131 = property on="Update Stage Pos" class="Bool (strict)"(error in=w239, "Val(Sgnl)"=FALSE ("Value (Signaling)")) -> (error out=w238:errorcluster)  [unwired: 1 in, 1 out]
      }
      event "Z Position": Value Change {
        # "TODO: Dont Know the Z Range. Check and Edit this part"
        n132 = event-data() -> ("NewVal"=w263:dbl)  [unwired: 1 in, 5 out]
        n133 = In Range and Coerce(upper limit=1.0, x=w263, lower limit=0.0) -> (coerced(x)=w259:dbl)  [unwired: 1 out]
        n134 = Multiply(x=10000.0, y=w259) -> (x*y=w258:dbl)
        n135 = call "Move Axis to Position.vi"("Position [internal units]"=w258, "Axis"=Axis_Name."Z", "VISA in"=w260) -> ("error out"=w254:errorcluster)  [unwired: 6 in, 1 out]
        n136 = property on="Update Stage Pos" class="Bool (strict)"(error in=w254, "Val(Sgnl)"=TRUE ("Value (Signaling)")) -> (error out=w252:errorcluster)  [unwired: 1 in, 1 out]
        n137 = property on="Update Stage Pos" class="Bool (strict)"(error in=w252, "Val(Sgnl)"=FALSE ("Value (Signaling)")) -> (error out=w251:errorcluster)  [unwired: 1 in, 1 out]
      }
    }
  }
  n138 = while {
    tunnel: w5 -> [w265]
    stop <- FALSE stop-if-true
    # "Direct Serial Communication with Stage"
    n139 = event shown="[0] \"Debug Mode\": Value Change" {
      selector: _ -> [_]
      dyn-events: _ -> [_]
      timeout: _ -> [_]
      tunnel: w265 -> [w266]
      event "Debug Mode": Value Change {
        # "Debug Mode directly \nhandles the commands\nand the Raw response \nis shown"
        n140 = event-data() -> ()  [unwired: 1 in, 6 out]
        n141 = case shown="True" "Debug Mode" {
          tunnel: w266 -> [_ w268]
          frame False {
          }
          frame True {
            n142 = while {
              tunnel: w268 -> [w271]
              stop <- FALSE stop-if-true
              n143 = event shown="[0] \"SendCommand To Stage\": Value Change" {
                selector: _ -> [_ _]
                dyn-events: _ -> [_ _]
                timeout: 0 -> [_ _]
                tunnel: w271 -> [w275 _]
                tunnel: [w272 _] -> _
                event "SendCommand To Stage": Value Change {
                  n144 = event-data() -> ()  [unwired: 1 in, 6 out]
                  n145 = call "Send Serial Command.vi"("Command"="Command", "VISA in"=w275) -> ("error out"=w272:errorcluster, "Response"=→"Response":string)  [unwired: 7 in, 1 out]
                }
                event Timeout {
                  n146 = event-data() -> ()  [unwired: 1 in, 3 out]
                }
              }
            }
          }
        }
      }
    }
  }
  n147 = while {
    tunnel: w5 -> [w278]
    i -> [w276]
    stop <- FALSE stop-if-true
    # "Use Position as the Start point"
    n148 = event shown="[1] \"Use Current Position as Start\": Value Change" {
      selector: _ -> [_ _]
      dyn-events: _ -> [_ _]
      timeout: _ -> [_ _]
      tunnel: w278 -> [_ w281]
      event Timeout {
        n149 = event-data() -> ()  [unwired: 1 in, 3 out]
      }
      event "Use Current Position as Start": Value Change {
        n150 = event-data() -> ("NewVal"=w282:bool)  [unwired: 1 in, 5 out]
        n151 = case shown="True" w282 {
          tunnel: w281 -> [_ w292]
          frame False {
            w288 = T10."Enabled" ("Disabled")
            n152 = property on="Start X" class="DigNum (strict)"("DisabledEnum"=w288) -> (error out=w285:errorcluster)  [unwired: 2 in, 1 out]
            n153 = property on="Start Y" class="DigNum (strict)"(error in=w285, "DisabledEnum"=w288) -> (error out=w284:errorcluster)  [unwired: 1 in, 1 out]
            n154 = property on="Stop X" class="DigNum (strict)"(error in=w284, "Caption.Text"="Stop X" ("Label.Text")) -> (error out=w283:errorcluster)  [unwired: 1 in, 1 out]
            n155 = property on="Stop Y" class="DigNum (strict)"(error in=w283, "Caption.Text"="Stop Y" ("Label.Text")) -> ()  [unwired: 1 in, 2 out]
          }
          frame True {
            w308 = T10."Disabled and Grayed Out" ("Disabled")
            n156 = property on="Start X" class="DigNum (strict)"("DisabledEnum"=w308) -> (error out=w307:errorcluster)  [unwired: 2 in, 1 out]
            n157 = property on="Start Y" class="DigNum (strict)"(error in=w307, "DisabledEnum"=w308) -> (error out=w291:errorcluster)  [unwired: 1 in, 1 out]
            n158 = call "Send Serial Command.vi"("Listen for response (T)"=TRUE, "error in (no error)"=w291, "Command"="ZERO", "VISA in"=w292) -> ("error out"=w289:errorcluster)  [unwired: 5 in, 2 out]
            n159 = property on="Update Stage Pos" class="Bool (strict)"(error in=w289, "Val(Sgnl)"=TRUE ("Value (Signaling)")) -> (error out=w295:errorcluster)  [unwired: 1 in, 1 out]
            n160 = property on="Update Stage Pos" class="Bool (strict)"(error in=w295, "Val(Sgnl)"=FALSE ("Value (Signaling)")) -> (error out=w294:errorcluster)  [unwired: 1 in, 1 out]
            n161 = property on="X Position" class="DigNum (strict)"(error in=w294) -> (error out=w304:errorcluster, "Value"=w306:dbl)  [unwired: 1 in, 1 out]
            n162 = property on="Start X" class="DigNum (strict)"(error in=w304, "Value"=w306) -> (error out=w303:errorcluster)  [unwired: 1 in, 1 out]
            n163 = property on="Y Position" class="DigNum (strict)"(error in=w303) -> (error out=w302:errorcluster, "Value"=w305:dbl)  [unwired: 1 in, 1 out]
            n164 = property on="Start Y" class="DigNum (strict)"(error in=w302, "Value"=w305) -> (error out=w298:errorcluster)  [unwired: 1 in, 1 out]
            n165 = property on="Stop X" class="DigNum (strict)"(error in=w298, "Caption.Text"="X Length (mm)" ("Label.Text")) -> (error out=w299:errorcluster)  [unwired: 1 in, 1 out]
            n166 = property on="Stop Y" class="DigNum (strict)"(error in=w299, "Caption.Text"="Y Length (mm)" ("Label.Text")) -> ()  [unwired: 1 in, 2 out]
          }
        }
      }
    }
    n167 = Equal To 0?(x=w276) -> (x = 0?=w277:bool)
    n168 = case shown="True" w277 {
      frame False {
      }
      frame True {
        # "This Executes the event atleast once"
        n169 = property on="Use Current Position as Start" class="Bool (strict)"("Val(Sgnl)"=FALSE ("Value (Signaling)")) -> ()  [unwired: 2 in, 2 out]
      }
    }
  }
  n170 = while {
    tunnel: [w309] -> w7
    stop <- FALSE stop-if-true
    # "Save Additional Data"
    n171 = event shown="[0] \"Setup Additional Data\": Value Change" {
      selector: _ -> [_]
      dyn-events: _ -> [_]
      timeout: _ -> [_]
      tunnel: ["Setup Additional Data"] -> _
      tunnel: [w311] -> w309
      event "Setup Additional Data": Value Change {
        w313 = TRUE ("Additional Data Set?")
        # "Add Additional Properties needed to be stored as attributes"
        n172 = event-data() -> ()  [unwired: 1 in, 6 out]
        n173 = call <vilib>:"Set Busy.vi"() -> ("error out"=w317:errorcluster)  [unwired: 10 in, 1 out]
        n174 = call "AdditionalInfoManupulation.vi"("error in"=w317, "Temperature"="Temperature") -> ("error out"=w316:errorcluster, "Additional Info"=w314:T4)  [unwired: 8 in]
        "Additional Info" <- w314
        n175 = call <vilib>:"Unset Busy.vi"("error in (no error)"=w316) -> ()  [unwired: 10 in, 1 out]
        n176 = Bundle("Additional Info"=w314, "Additional Data Set?"=w313) -> (w312:T13)  [unwired: 1 in]
        n177 = call <extravilib>:"Write.vi"("element"=w312) -> ("channel"=w311:T14)  [unwired: 1 out]
        "Additional Data Set?" <- w313
      }
    }
  }
  n178 = while {
    tunnel: [w319] -> w2
    stop <- FALSE stop-if-true
    # "Generator Setup"
    n179 = event shown="[0] \"Setup Generator\": Value Change" {
      selector: _ -> [_]
      dyn-events: _ -> [_]
      timeout: _ -> [_]
      tunnel: [w324] -> w319
      event "Setup Generator": Value Change {
        n180 = event-data() -> ()  [unwired: 1 in, 6 out]
        n181 = call <vilib>:"Set Busy.vi"() -> ("error out"=w330:errorcluster)  [unwired: 10 in, 1 out]
        n182 = call "InitGenerator.vi"("error in (no error)"=w330, "Generator ID in"="Generator ID") -> ("error out"=w329:errorcluster, "Init Done"=w328:bool, "Waveform"=→"Input Graph":cluster{"tv":dbl[], "DAC Codes":u16[]}, "Generator Info"=w323:T7)  [unwired: 5 in, 1 out]
        "Generator Info" <- w323
        n183 = call <vilib>:"Unset Busy.vi"("error in (no error)"=w329) -> ("error out"=w332:errorcluster)  [unwired: 10 in]
        n184 = Unbundle By Name(w332) -> ("status"=w327:bool)
        n185 = Compound Arithmetic op=AND(w328, invert w327, "Setup Generator") -> (w322:bool)
        "Generator Ready?" <- w322
        n186 = Bundle("Generator Info"=w323, w322) -> (w321:cluster{"Generator Info":T7, bool})  [unwired: 1 in]
        n187 = call <extravilib>:"Write.vi"("element"=w321) -> ("channel"=w324:T15)  [unwired: 1 out]
      }
    }
  }
  n188 = while {
    tunnel: [w333] -> w1
    stop <- FALSE stop-if-true
    # "Digitizer Setup"
    n189 = event shown="[0] \"Setup Digitizer\": Value Change" {
      selector: _ -> [_]
      dyn-events: _ -> [_]
      timeout: _ -> [_]
      tunnel: [w338] -> w333
      event "Setup Digitizer": Value Change {
        n190 = event-data() -> ()  [unwired: 1 in, 6 out]
        n191 = call <vilib>:"Set Busy.vi"() -> ()  [unwired: 10 in, 2 out]
        n192 = call "InitDigitizer.vi"("Digitizer ID"="Digitizer ID", "Delay After Trig (us)"="Delay after Trigger (us)", "Sampling Frequency"="Sampling Rate (Fs)", "Trigger Type"="Trigger Type", "Record Size"="Record Size (Samples)", "Trigger Level (V)"="Trigger Level (V)") -> ("TIS Configured?"=w347:bool, "Clocking Configured?"=w346:bool, "Default Configured?"=w345:bool, "Digitizer Info"=w336:T5, "Error out"=w348:errorcluster)  [unwired: 5 in]
        "TIS Configured?" <- w347
        "Clocking Option Configured?" <- w346
        "Default Configured?" <- w345
        "Digitizer Info" <- w336
        n193 = Compound Arithmetic op=AND(w347, w346, w345, "Setup Digitizer") -> (w335:bool)
        "Digitizer Configured?" <- w335
        n194 = call <vilib>:"Unset Busy.vi"("error in (no error)"=w348) -> ()  [unwired: 10 in, 1 out]
        n195 = Bundle("Digitizer Info"=w336, w335) -> (w337:cluster{"Digitizer Info":T5, bool})  [unwired: 1 in]
        n196 = call <extravilib>:"Write.vi"("element"=w337) -> ("channel"=w338:T16)  [unwired: 1 out]
      }
    }
  }
  n197 = while {
    stop <- FALSE stop-if-true
    # "Gating Cursors Control"
    n198 = event shown="[0] \"Output Graph\": Cursor Move" {
      selector: _ -> [_ _]
      dyn-events: _ -> [_ _]
      timeout: _ -> [_ _]
      event "Output Graph": Cursor Move {
        n199 = event-data() -> ("CursIdx"=w352:i32, "CursLoc"=w351:cluster{"X":dbl, "Y":dbl})  [unwired: 1 in, 7 out]
        n200 = case shown="1" w352 {
          tunnel: w351 -> [w354 w358]
          frame 0, Default {
            n201 = Unbundle By Name(w354) -> ("X"=w353:dbl)
            n202 = property on="Start Depth" class="DigNum (strict)"("Value"=w353) -> ()  [unwired: 2 in, 2 out]
          }
          frame 1 {
            n203 = Unbundle By Name(w358) -> ("X"=w355:dbl)
            n204 = property on="Start Depth" class="DigNum (strict)"() -> ("Value"=w357:dbl)  [unwired: 2 in, 2 out]
            n205 = Subtract(x=w355, y=w357) -> (x-y=w356:dbl)
            n206 = property on="Length" class="DigNum (strict)"("Value"=w356) -> ()  [unwired: 2 in, 2 out]
          }
        }
      }
      event "Start Depth", "Length": Value Change {
        n207 = event-data() -> ()  [unwired: 1 in, 6 out]
        n208 = property on="Output Graph" class="WFGraph (strict)"("Active Cursor"=u32 0) -> (error out=w368:errorcluster)  [unwired: 2 in, 1 out]
        n209 = property on="Start Depth" class="DigNum (strict)"(error in=w368) -> (error out=w367:errorcluster, "Value"=w369:dbl)  [unwired: 1 in, 1 out]
        n210 = property on="Output Graph" class="WFGraph (strict)"(error in=w367, "Cursor.Cursor X"=w369) -> (error out=w364:errorcluster)  [unwired: 1 in, 1 out]
        n211 = property on="Output Graph" class="WFGraph (strict)"(error in=w364, "Active Cursor"=u32 1) -> (error out=w366:errorcluster)  [unwired: 1 in, 1 out]
        n212 = property on="Start Depth" class="DigNum (strict)"(error in=w366) -> (error out=w360:errorcluster, "Value"=w362:dbl)  [unwired: 1 in, 1 out]
        n213 = property on="Length" class="DigNum (strict)"(error in=w360) -> (error out=w359:errorcluster, "Value"=w363:dbl)  [unwired: 1 in, 1 out]
        n214 = Add(x=w362, y=w363) -> (x+y=w361:dbl)
        n215 = property on="Output Graph" class="WFGraph (strict)"(error in=w359, "Cursor.Cursor X"=w361) -> ()  [unwired: 1 in, 2 out]
      }
    }
  }
  n216 = while {
    stop <- FALSE stop-if-true
    n217 = event shown="[0] \"Find Delay after Trig\": Value Change" {
      selector: _ -> [_]
      dyn-events: _ -> [_]
      timeout: _ -> [_]
      event "Find Delay after Trig": Value Change {
        n218 = event-data() -> ()  [unwired: 1 in, 6 out]
      }
    }
  }
  n219 = while {
    tunnel: w8 -> [w393]
    tunnel: w1 -> [w392]
    tunnel: w2 -> [w391]
    tunnel: w7 -> [w390]
    shift-right: [w385] -> _
    shift-left: _ -> [w378]
    shift-right: [w382] -> _
    shift-left: _ -> [w379]
    shift-right: [w383] -> _
    shift-left: _ -> [w380]
    shift-right: [w384] -> _
    shift-left: _ -> [w381]
    shift-right: [w377] -> _
    shift-left: _ -> [w375]
    shift-right: [w376] -> _
    shift-left: _ -> [w374]
    shift-right: [w372] -> _
    shift-left: ScanStates."idle" -> [w373]
    stop <- FALSE stop-if-true
    n220 = call <extravilib>:"Read.vi"("channel"=w391) -> ("element"=w388:cluster{"Generator Info":T7, bool})  [unwired: 1 in, 1 out]
    n221 = call <extravilib>:"Read.vi"("channel"=w392) -> ("element"=w387:cluster{"Digitizer Info":T5, bool})  [unwired: 1 in, 1 out]
    n222 = call <extravilib>:"Read.vi"("channel"=w393) -> ("element"=w386:cluster{"Stage Setup Info":T8, bool})  [unwired: 1 in, 1 out]
    n223 = call <extravilib>:"Read.vi"("channel"=w390) -> ("element"=w389:T13)  [unwired: 1 in, 1 out]
    n224 = case shown="\"scan\"" w373 {
      selector: w373 -> [w396 _ _ w583 w592]
      tunnel: [w409 ScanStates."scan" ScanStates."idle" w583 w592] -> w372
      tunnel: w389 -> [w413 _ _ _ _]
      tunnel: w388 -> [w412 _ _ _ _]
      tunnel: w387 -> [w411 _ _ _ _]
      tunnel: w386 -> [w410 _ _ _ _]
      tunnel: [w402 w417 w474 w578 w591] -> w384
      tunnel: [w401 w416 w470 w577 w590] -> w383
      tunnel: [w400 w421 w476 w582 w589] -> w382
      tunnel: [w399 w418 w473 w581 w588] -> w385
      tunnel: w381 -> [_ w417 w474 w578 w591]
      tunnel: w380 -> [_ w416 w470 w577 w590]
      tunnel: w379 -> [_ w421 w476 w582 w589]
      tunnel: w378 -> [_ w418 w473 w581 w588]
      tunnel: [w398 w420 w475 w580 w585] -> w377
      tunnel: [w397 w419 w471 w579 w584] -> w376
      tunnel: w375 -> [w398 _ w475 w580 w585]
      tunnel: w374 -> [w397 _ w471 w579 w584]
      frame "idle", Default {
        n225 = Unbundle(w412) -> ("Generator Info"=w402:T7, w408:bool)
        n226 = Unbundle(w411) -> ("Digitizer Info"=w401:T5, w407:bool)
        n227 = Unbundle(w410) -> ("Stage Setup Info"=w399:T8, w406:bool)
        n228 = Unbundle(w413) -> ("Additional Info"=w400:T4, "Additional Data Set?"=w405:bool)
        n229 = Compound Arithmetic op=AND(w408, w407, w406, w405, "Setup Scan") -> (w403:bool)
        n230 = Select(t=ScanStates."init", s=w403, f=w396) -> (s? t:f=w409:T1)
      }
      frame "init" {
        # "Open File With the attr"
        # "Arm"
        n231 = call "OpenH5WithAttr.vi"("Filename"="Filename", "Additional Info"=w421, "File Directory"="File Directory", "Generator Info"=w417, "Digitizer Info"=w416, "Stage Setup Info"=w418) -> ("error out"=w428:errorcluster, "HDF5 Ref out"=w427:T18)  [unwired: 4 in]
        n232 = xnode "Simple OpenCreateReplace Dataset"("Dataset Path"="data", "HDF5 Ref"=w427, "Unlimited  dataset (F)"=TRUE, "error in (no error)"=w428, "operation"=LVH5D_Operation."create or replace", "Datatype and Dataspace"=u64[][] [] ("appended array")) -> ("HDF5 Dataset Ref out"=w419:T18, "HDF5 Ref out"=w420:T18)  [unwired: 2 in, 1 out]
        n233 = call "ArmDevices.vi"("Digitizer Info"=w416, "Generator Info"=w417) -> ()  [unwired: 3 in, 3 out]
      }
      frame "scan" {
        n234 = Unbundle By Name(w473) -> ("X Pixels Count"=w440:i32, "Y Lines Count"=w443:i32, "Scan Mode"=w454:enum16{"Raster Scan", "Serpentine Scan"})
        n235 = Unbundle By Name(w474) -> ("Generator ID"=w462:T6)
        n236 = call "GetFPGA1212Reference.vi"("RIO Device IN"=w462) -> ("error out"=w465:errorcluster, "FPGA VI Reference Out"=w464:refnum<k20>)  [unwired: 1 in]
        n237 = xnode "Read/Write Control"("FPGA VI Reference In"=w464, "error in"=w465, "Vi_Trig/nStage_Trig"=FALSE ("Trig In")) -> ("FPGA VI Reference Out"=w467:refnum<k20>, "error out"=w466:errorcluster)
        n238 = Unbundle By Name(w473) -> ("Stage Visa"=w461:refnum<visa-resource-name>)
        n239 = xnode "Close FPGA VI Reference"("FPGA VI Reference In"=w467, "error in"=w466) -> ("error out"=w457:errorcluster)
        n240 = call "Send Serial Command.vi"("Listen for response (T)"=TRUE, "error in (no error)"=w457, "Command"="SCAN", "VISA in"=w461) -> ("error out"=w459:errorcluster, "Response"=w458:string)  [unwired: 5 in, 1 out]
        n241 = call "Parse Serial Response.vi"("error in (no error)"=w459, "Raw Response"=w458) -> ("error out"=w455:errorcluster)  [unwired: 6 in, 3 out]
        n242 = Unbundle By Name(w470) -> ("Digitizer ID"=w452:T6, "Number of Elements"=w450:u16)
        n243 = property on="Update Stage Pos" class="Bool (strict)"(error in=w455, "Val(Sgnl)"=TRUE ("Value (Signaling)")) -> (error out=w451:errorcluster)  [unwired: 1 in, 1 out]
        n244 = call "Get5772Ref.vi"("error in (no error)"=w451, "RIO Device IN"=w452) -> ("FPGA VI Reference Out"=w449:refnum<k20>)  [unwired: 1 out]
        n245 = while {
          tunnel: [w501] -> w472
          tunnel: w440 -> [w490]
          tunnel: w443 -> [w489]
          tunnel: w454 -> [w487]
          tunnel: w449 -> [w500]
          tunnel: w450 -> [w498]
          tunnel: [w496] -> w448
          shift-right: [w494] -> _
          shift-left: 0 -> [w495]
          stop <- w488 stop-if-true
          # "Fetch Data From Digitizer"
          n246 = stacked-sequence {
            tunnel: w500 -> [w515 _]
            tunnel: [w513 _] -> w499
            tunnel: w498 -> [w512 _]
            tunnel: [w504 _] -> w497
            tunnel: [w503 _] -> w496
            tunnel: w495 -> [_ w527]
            tunnel: [_ w523] -> w494
            tunnel: [_ w519] -> w493
            tunnel: [_ w518] -> w491
            tunnel: w490 -> [_ w517]
            tunnel: w489 -> [_ w525]
            tunnel: [_ w522] -> w488
            tunnel: w487 -> [_ w521]
            frame #0 {
              n247 = xnode "Invoke Method"("FPGA VI Reference In"=w515, "Number of Elements"=w512, "Timeout (ms)"=8000) -> ("FPGA VI Reference Out"=w503:refnum<k20>, "Data"=w502:u64[])  [unwired: 1 in, 2 out]
              n248 = Split Number(x=w502) -> (hi(x)=w505:u32[], lo(x)=w506:u32[])
              n249 = Array Size(array=w502) -> (size(s)=w511:i32)
              n250 = Split Number(x=w505) -> (hi(x)=w507:u16[], lo(x)=w510:u16[])
              n251 = Split Number(x=w506) -> (hi(x)=w509:u16[], lo(x)=w508:u16[])
              n252 = Interleave 1D Arrays(w507, w510, w509, w508) -> (w504:u16[])
              n253 = Equal?(x=w512, y=w511) -> (x = y?=w513:bool)
            }
            frame #1 {
              n254 = Increment(x=w527) -> (x+1=w523:i32)
              n255 = Multiply(x=w517, y=w525) -> (x*y=w524:i32)
              n256 = Equal?(x=w523, y=w524) -> (x = y?=w522:bool)
              n257 = Quotient & Remainder(x=w523, y=w517) -> (floor(x/y)=w518:i32)  [unwired: 1 out]
              n258 = Multiply(x=w517, y=w518) -> (x*y=w526:i32)
              n259 = Subtract(x=w523, y=w526) -> (x-y=w520:i32)
              n260 = Decrement(x=w520) -> (x-1=w516:i32)
              n261 = case shown="\"Serpentine Scan\"" w521 {
                tunnel: w516 -> [w528 w531]
                tunnel: [w528 w529] -> w519
                tunnel: w518 -> [_ w536]
                tunnel: w517 -> [_ w534]
                frame "Raster Scan", Default {
                }
                frame "Serpentine Scan" {
                  n262 = Quotient & Remainder(x=w536, y=2) -> (x-y*floor(x/y)=w533:i32)  [unwired: 1 out]
                  n263 = Multiply(x=w534, y=w533) -> (x*y=w532:i32)
                  n264 = Subtract(x=w532, y=w531) -> (x-y=w530:i32)
                  n265 = Absolute Value(x=w530) -> (abs(x)=w529:i32)
                }
              }
            }
          }
          n266 = Bundle(w493, w491, w497) -> (w492:cluster{i32, i32, u16[]})  [unwired: 1 in]
          n267 = call <extravilib>:"Write.vi"("last element? (F)"=w488, "element"=w492, "element valid? (T)"=w499) -> ("channel"=w501:T19)  [unwired: 6 in, 2 out]
        }
        n268 = xnode "Close FPGA VI Reference"("FPGA VI Reference In"=w448) -> ()  [unwired: 1 in, 1 out]
        n269 = Unbundle By Name(w470) -> ("Sampling Frequency"=w469:dbl, "range (Vpp)"=w468:dbl)
        n270 = Initialize Array(u32 0 ("element"), w443, w440) -> (w441:u32[][])
        n271 = Initialize Array(0.0 ("element"), w443, w440) -> (w442:dbl[][])
        n272 = while {
          tunnel: w472 -> [w568]
          tunnel: w471 -> [w540]
          tunnel: w469 -> [w538]
          tunnel: w468 -> [w565]
          shift-right: [w542] -> _
          shift-left: w442 -> [w556]
          shift-right: [w548] -> _
          shift-left: w441 -> [w555]
          stop <- w567 stop-if-true
          # "Post Process Data"
          n273 = call <extravilib>:"Read.vi"("channel"=w568) -> ("last element?"=w567:bool, "element"=w566:T20)  [unwired: 6 in, 3 out]
          n274 = Unbundle By Name(w566) -> ("X Pixel"=w553:i32, "Y Pixel"=w554:i32, "Data"=w537:u64[])
          n275 = Build Array(w537) -> (w541:u64[][])
          n276 = xnode "Append Element(s) to Dataset"("HDF5 Dataset Ref"=w540, "Data Element(s)"=w541) -> ()  [unwired: 2 in, 4 out]
          n277 = call "Scale Acquired Data.vi"("range (V)"=w565, "Sample Rate"=w538, "Number of Bits"=i16 12, "Data In"=w537) -> ("output waveform"=w559:waveform(ext))  [unwired: 7 out]
          n278 = Unbundle By Name(w559) -> ("dt"=w558:dbl, "Y"=w557:ext[])
          n279 = call <vilib>:"Fast Hilbert Transform.vi"("X"=w557) -> ("Hilbert{X}"=w563:dbl[])  [unwired: 1 out]
          n280 = Complex To Polar(r * e^(i*theta)=w563) -> (r=w552:dbl[])  [unwired: 1 out]
          n281 = Array Max & Min(array=w552) -> (max value=w551:dbl, max index (indices)=w550:i32)  [unwired: 2 out]
          n282 = Build Array(w557, w552) -> (w562:ext[][])
          n283 = Replace Array Subset(array=w555, new element=w550, index (row)=w554, index (col)=w553) -> (w548:u32[][])
          n284 = Replace Array Subset(array=w556, new element=w551, index (row)=w554, index (col)=w553) -> (w542:dbl[][])
          n285 = Bundle(0.0, "dt"=w558, w562) -> (→"Output Graph":cluster{dbl, "dt":dbl, ext[][]})  [unwired: 1 in]
          n286 = call "FrequencyResponse.vi"("DAC Codes"=w537, "Sampling Frequency (Hz)"=w538) -> ("Frequency Response"=→"Output Graph FFT":cluster{dbl[], dbl[]})  [unwired: 8 in, 1 out]
          n287 = call-poly <vilib>:"Plot Helper.vi"("z matrix"=w548) -> ("3D Plot lvclass Array out"=→"3D Mesh":refnum<class "3D Plot Datatype.lvclass">[])  [unwired: 5 in, 5 out]
          n288 = control-ref of="Image"() -> (w547:refnum<vi>)
          n289 = call "DisplayImagePlot.vi"("Data Array"=w542, "Picture For Size Ref"=w547, "Colormap"="Colorbar", "Axis"="Axis", "Map"="Colormap") -> ("Picture"=→"Image":picture)  [unwired: 6 in]
        }
        n290 = disable-structure shown="Disabled" {
          frame Disabled {
            n291 = case shown="False" "Data Gating" {
              tunnel: [u32 0 ("Start Depth") w483] -> _
              tunnel: [u32 5000 ("Length") w484] -> _
              tunnel: _ -> [_ w480]
              frame False {
              }
              frame True {
                n292 = Multiply(x=w480, y="Start Depth") -> (x*y=w481:dbl)
                n293 = Multiply(x=w480, y="Length") -> (x*y=w482:dbl)
                n294 = To Unsigned Long Integer(number=w481) -> (unsigned 32bit integer=w483:u32)
                n295 = To Unsigned Long Integer(number=w482) -> (unsigned 32bit integer=w484:u32)
              }
            }
          }
          frame Enabled {
          }
        }
      }
      frame "endscan" {
        n296 = call "DisArmDevices.vi"("Digitizer Info"=w577, "Generator Info"=w578) -> ()  [unwired: 3 in, 3 out]
      }
      frame "closefiles" {
        w586 = TRUE ("Force Close (F)")
        n297 = call <vilib>:"H5Dclose.vi"("HDF5 Dataset Ref"=w584) -> ("error out"=w587:errorcluster)  [unwired: 8 in]
        n298 = call <vilib>:"H5Fclose.vi"("error in (no error)"=w587, "Force Close (F)"=w586, "Close All Open Objects (T)"=w586, "HDF5 Ref"=w585) -> ()  [unwired: 5 in, 1 out]
      }
    }
    "State" <- w373
  }
